vi "STED Control V18 DL.vi"() -> ()   [LabVIEW 2014]
uses:
  Controls/Button 2.ctl
  Type Defs/Image Acquisition Parameters.ctl
  Laser Controls.ctl
  Detectors.ctl
  Type Defs/P541.ctl
  Type Defs/M227.ctl
  Type Defs/P612.ctl
  Type Defs/M686.ctl
  Type Defs/P841.ctl
  Type Defs/ASI.ctl
  Type Defs/N664_V2.ctl
  Type Defs/STED Graph Controls.ctl
  Type Defs/Display Controls.ctl
  Type Defs/Z comp.ctl
  FPGA-7842R-Reference.ctl
  Manual Controls V2.ctl
  Scan Parameters.ctl
  <vilib>/Utility/miscctls.llb/LVPositionTypeDef.ctl
  Controls/StageStates.ctl
  DM_Dual_V2/Controls/Standard Action.ctl
  Focus Lock/Controls/Counter Action.ctl
  Focus Lock/Controls/Standard Action for Focus Lock.ctl
  <vilib>/Utility/miscctls.llb/LVRectTypeDef.ctl
  <vilib>/event_ctls.llb/lveventtype.ctl
  <vilib>/Utility/file.llb/Read From Spreadsheet File (DBL).vi
  <vilib>/FPGAPlugInAG/PCIe-7841R/niLvFpga_Open_PCIe-7841R.vi
  <vilib>/FPGAPlugInAG/PCIe-7841R/niLvFpga_Abort_PCIe-7841R.vi
  <vilib>/Utility/file.llb/Write To Spreadsheet File (DBL).vi
  <vilib>/rvi/interface/nirviOpenFPGA/nirviOpenFPGA.xnode
  FPGA Bitfiles/MainSTEDFPGAProj_FPGATarget_WaveformandLaser_sIm2Xng7ncM.lvbitx
  FPGA Target VIs/FPGA-7841R/Waveform and Laser Controls V7.vi
  <vilib>/rvi/interface/nirviMethod/nirviMethod.xnode
panel:
  in  "Wake Up FPGA":bool
  in  "z Comp.":T1
  out "Graph Ref Out":refnum<vi>[](array[refnum])
  out "Frame Counter":i32
  in  "Follow Cursor":bool
  in  "Laser Controls 2":T2={"Laser On Time (Ticks)"=16, "Laser Delay (Ticks)"=3}
  out "Channel 6":sgl[][](graph)
  out "Channel 5":sgl[][](graph)
  out "Channel 4":sgl[][](graph)
  out "Channel 3":sgl[][](graph)
  out "Channel 2":sgl[][](graph)
  out "Channel 1":sgl[][](graph)
  in  "Display Controls":T3
  in  "Graph Tools":T4={"Zoom Out"=FALSE, "Zoom In"=FALSE, "Reset Zoom"=FALSE, "Pan Tool"=FALSE, "Show Cursor"=FALSE, "Load File"=FALSE, "Fit Tool"=FALSE, "Smooth Tool"=FALSE, "Merge Tool"=FALSE, "Auto Scale"=FALSE, "Apply Color"=FALSE, "Color Map"=enum."Fire"}
  in  "Shutters":T5
  in  "Upper Objective Z - N664":T6={"Up N664"=FALSE, "Down N664"=FALSE, "Step Size (um)"=0.001, "Position (mm)"=0.0, "Home"=FALSE, "Save"=FALSE} {"Step Size (um)" min=0.001}
  in  "Cavity Translation Z - ASI":T7={"Up ASI"=FALSE, "Down ASI"=FALSE, "Step Size (um)"=0.001, "Z (um)"=0.001, "F (um)"=0.001, "Velocity"=0.001} caption="ASI" {"Velocity" min=0.001; "F (um)" min=0.001; "Z (um)" min=-1500.0 max=1500.0; "Step Size (um)" min=0.001}
  in  "Phase Comp Mirror - P841":T8={"Position (µm)"=0.0, "Step Size (µm)"=0.05, "Up P841"=FALSE, "Down P841"=FALSE}
  in  "Sample Stage XY - M686":T9={"Home Button"=FALSE, "Left Button"=FALSE, "Down Button"=FALSE, "Right Button"=FALSE, "Up Button"=FALSE, "X"=0.0, "Y"=0.0, "Step Size (um)"=1.0} {"Y" format="%#_8g"; "X" format="%#_8g"}
  in  "Bottom Objective XY - P612":T10
  in  "Abort AllStage":bool
  in  "Stages":T11={"M227"=TRUE, "N664"=TRUE, "P612"=TRUE, "M686"=TRUE, "P841"=TRUE, "ASI"=FALSE}
  in  "Sample Z Coarse - M227":T12
  in  "Tab Control":T13(tab)
  in  "SLM":T14
  in  "DM":T14
  in  "Timing":T14
  in  "Focus Lock":T14
  in  "Sequence":T14
  in  "Stage Monitor":T14
  in  "Camera":T14
  in  "Sequence Cluster":T15
  in  "Sample Z - P541":T16={"Step Up"=FALSE, "Step Down"=FALSE, "Z Position"=0.0, "Step Size (um)"=1.0, "Home"=FALSE, "Save"=FALSE}
  in  "Detectors":T17={"PMT"=TRUE, "Far Red (685/40 nm)"=FALSE, "Orange (624/40 nm)"=FALSE, "Green (525/50 nm)"=FALSE, "Sum All"=FALSE}
  in  "Laser Controls":T18 {"STED Power (V)" scale=0.0..10.0}
  in  "Save File Path":path=path "C:/isoSTED_Data/Temp/Test_0000.dbl"
  in  "Capture":bool
  in  "Image Acquisition Parameters":T19={"Scan Type"=enum."Beam Scanning", "Scan Mode"=enum."XY", "Fast Axis Frequency (Hz)"=15780.0, "Image Format"=256, "Line Accumulations"=100, "Frames Per Capture"=1, "Frames Accumulations"=1, "Image Dimension (um)"=[15.0, 15.0], "Number of Z Steps"=1, "Z Steps Size (um)"=1.0, "Pixel Size (nm)"=[58.59375, 58.59375], "Customized Image Format"=[]} {"Z Steps Size (um)" min=0.0; "Number of Z Steps" min=1; "Frames Accumulations" min=1; "Frames Per Capture" min=1; "Line Accumulations" min=1; "Image Format" items=["64 x 64"=64, "128 x 128"=128, "256 x 256"=256, "512 x 512"=512, "1024 x 1024"=1024, "2048 x 2048"=2048, "Customized..."=0]}
  in  "Live":T14
  in  "Exit":bool
  # "Piston"
  # "Defocus"
  # "Spherical"
  # "Frame Mode"
  # "Line Mode"
  # "Length"
  # "Height"
  # "XY"
  # "Z"
  # "Length"
  # "Height"
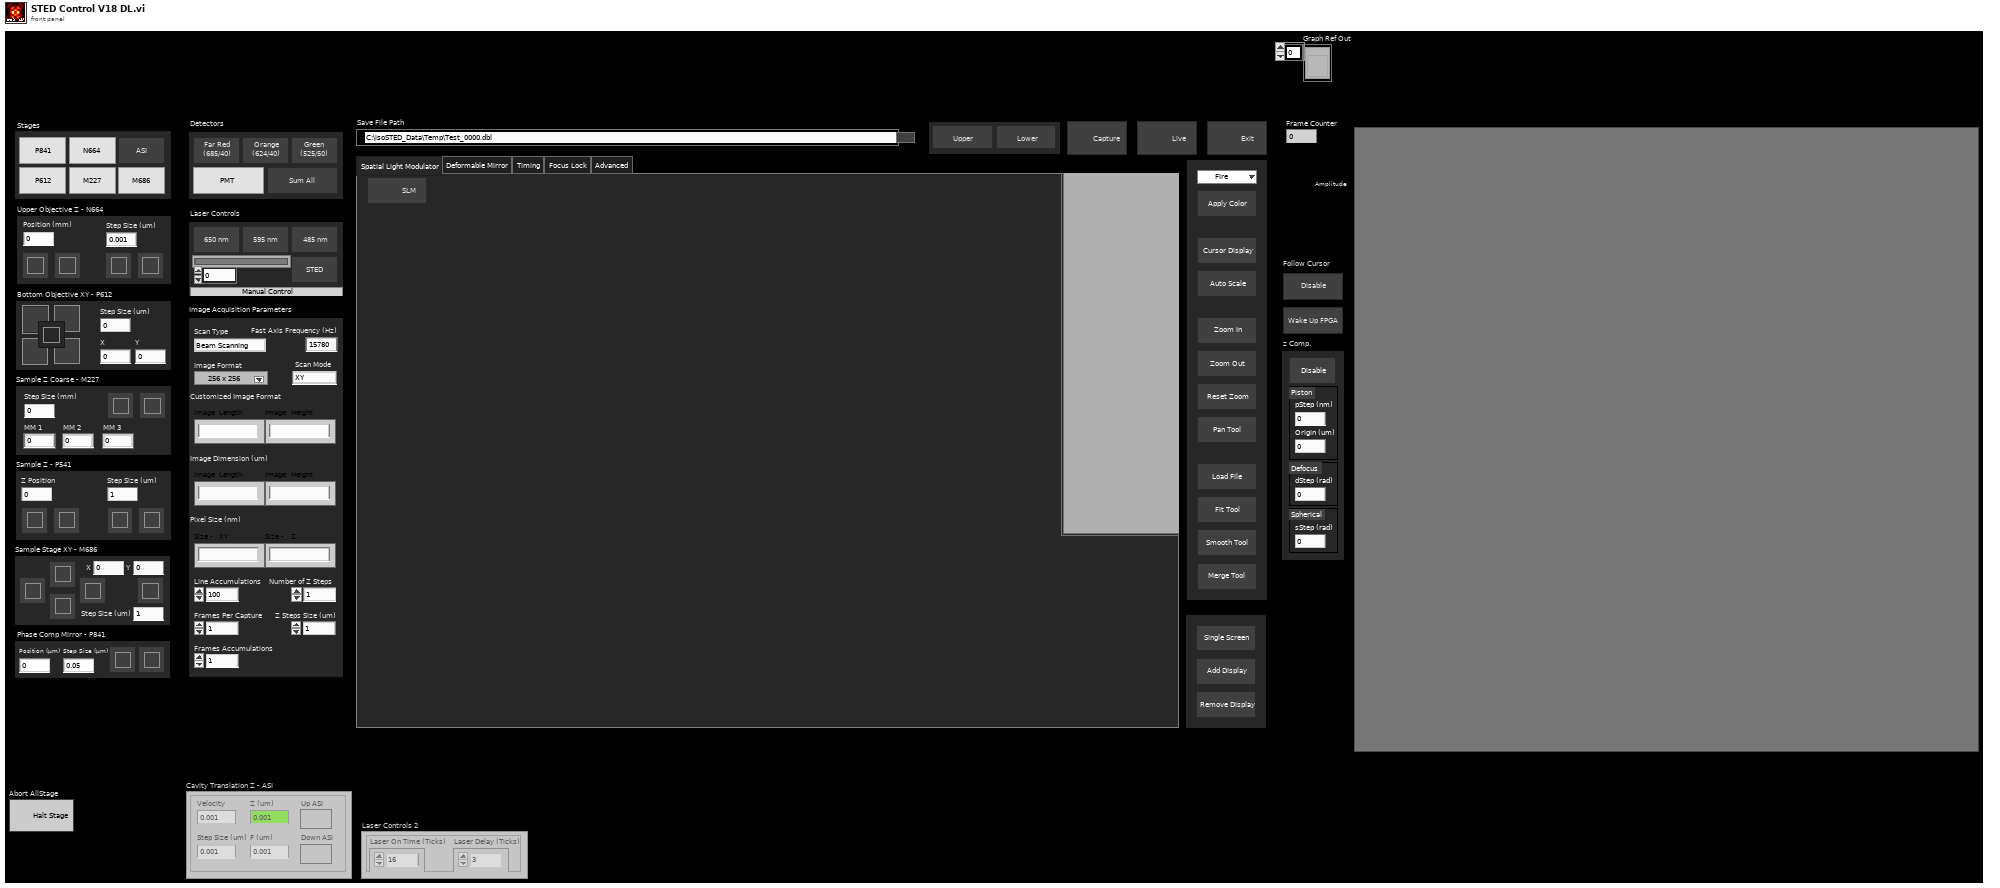
[diagram p1: front panel]
types:
  T1 = typedef "Z comp.ctl" = cluster{"Enable":bool, "pStep (nm)":dbl, "Origin (um)":dbl, "dStep (rad)":dbl, "sStep (rad)":dbl}
  T2 = cluster{"Laser On Time (Ticks)":i8, "Laser Delay (Ticks)":i8}
  T3 = typedef "Display Controls.ctl" = cluster{"Remove Display":bool, "Add Display":bool, "Single Screen":bool}
  T4 = typedef "STED Graph Controls.ctl" = cluster{"Zoom Out":bool, "Zoom In":bool, "Reset Zoom":bool, "Pan Tool":bool, "Show Cursor":bool, "Load File":bool, "Fit Tool":bool, "Smooth Tool":bool, "Merge Tool":bool, "Auto Scale":bool, "Apply Color":bool, "Color Map":enum16{"System", "Fire", "Gray", "Red", "Green", "Blue", "Cyan", "Magenta", "Yellow", "Red-White", "Green-White", "Blue-White", "Glow"}}
  T5 = cluster{"Upper Shutter":bool, "Lower Shutter":bool}
  T6 = typedef "N664_V2.ctl" = cluster{"Up N664":bool, "Down N664":bool, "Step Size (um)":dbl, "Position (mm)":dbl, "Home":bool, "Save":bool}
  T7 = typedef "ASI.ctl" = cluster{"Up ASI":bool, "Down ASI":bool, "Step Size (um)":dbl, "Z (um)":dbl, "F (um)":dbl, "Velocity":dbl}
  T8 = typedef "P841.ctl" = cluster{"Position (µm)":dbl, "Step Size (µm)":dbl, "Up P841":bool, "Down P841":bool}
  T9 = typedef "M686.ctl" = cluster{"Home Button":bool, "Left Button":bool, "Down Button":bool, "Right Button":bool, "Up Button":bool, "X":dbl, "Y":dbl, "Step Size (um)":dbl}
  T10 = typedef "P612.ctl" = cluster{"Home Button":bool, "Up Button":bool, "Left Button":bool, "Down Button":bool, "Right Button":bool, "Step Size (um)":dbl, "X":dbl, "Y":dbl}
  T11 = cluster{"M227":bool, "N664":bool, "P612":bool, "M686":bool, "P841":bool, "ASI":bool}
  T12 = typedef "M227.ctl" = cluster{"Up M227":bool, "Down M227":bool, "Step Size (mm)":dbl, "MM 1":dbl, "MM 2":dbl, "MM 3":dbl}
  T13 = enum32{"Spatial Light Modulator", "Deformable Mirror", "Timing", "Focus Lock", "Advanced"}
  T14 = typedef "Button 2.ctl" = bool
  T15 = cluster{"Operation Option":enum32{"frameSeq", "lineSeq"}, "AddSeq":bool, "DeleteSeq":bool, "DeleteAllSeq":bool, "Sequence List":enum32{"Seq 1", "Seq 2", "Seq 3", "Seq 4"}}
  T16 = typedef "P541.ctl" = cluster{"Step Up":bool, "Step Down":bool, "Z Position":dbl, "Step Size (um)":dbl, "Home":bool, "Save":bool}
  T17 = typedef "Detectors.ctl" = cluster{"PMT":bool, "Far Red (685/40 nm)":bool, "Orange (624/40 nm)":bool, "Green (525/50 nm)":bool, "Sum All":bool}
  T18 = typedef "Laser Controls.ctl" = cluster{"STED Power (V)":dbl, "STED":bool, "650 nm":bool, "590 nm":bool, "485 nm":bool, "Manual Control":bool}
  T19 = typedef "Image Acquisition Parameters.ctl" = cluster{"Scan Type":enum16{"Sample Scanning", "Beam Scanning"}, "Scan Mode":enum16{"XY", "XZ", "YZ", "XYZ"}, "Fast Axis Frequency (Hz)":dbl, "Image Format":u16, "Line Accumulations":u16, "Frames Per Capture":u16, "Frames Accumulations":u16, "Image Dimension (um)":dbl[], "Number of Z Steps":u16, "Z Steps Size (um)":dbl, "Pixel Size (nm)":dbl[], "Customized Image Format":dbl[]}
  T20 = typedef "Scan Parameters.ctl" = cluster{"Fast_Ax_Amp_V":dbl, "Fast_Ax_Off_V":dbl, "Slow_Ax_Amp_V":dbl, "Slow_Ax_Off_V ":dbl, "Slow_Ax_Max_V_VperS":dbl, "Slow_Ax1_Del25ns":i32, "Slow_Ax2_Del25ns":i32, "Stage_X_Off_V":dbl, "Stage_Y_Off_V":dbl, "Stage_Z_Off_V":dbl, "Galvo1_Off_V":dbl, "Galvo2_Off_V":dbl, "Last_Scan_Mode":enum16{"XY", "XZ", "YZ", "XYZ"}, "Current_Scan_Mode":enum16{"XY", "XZ", "YZ", "XYZ"}, "Fly_Back_Lines":u16, "Linear_Ramp_End":u32, "Z_Step_I16":i16, "Z_Start_I16":i16, "Laser_States _U32":u32, "590_Voltage_I16":i16, "775_AOM_Volt_I16":i16, "Blanking OFF":bool, "Unused_Axis_I16":i16}
  T21 = typedef "Manual Controls V2.ctl" = cluster{"Galvo 1 Position (I16)":i16, "Galvo 2 Position (I16)":i16, "X Axis Voltage (I16)":i16, "Y Axis Voltage (I16)":i16, "Z Axis Voltage (I16)":i16, "Res Mirror Amp (I16)":i16, "Res Mirror Mute":bool, "Upper Shutter":bool, "Lower Shutter":bool}
  T22 = typedef "FPGA-7842R-Reference.ctl" = enum16{"Stage Control", "Laser Control", "Unused Axis I16", "Exit", "Set Res Mirror", "Set Galvo", "Current Frame for Capture", "Default", "Close FPGA", "Stop Waveforms", "Start Waveforms", "Shutter Control", "Initialize"}
  T23 = typedef "Counter Action.ctl" = enum16{"Zero", "Plus One", "Read"}
  T24 = typedef "StageStates.ctl" = enum16{"POSITION", "MVR", "MOVE", "HALT", "ONTARGET", "ERROR", "EXIT", "HOME", "ZEROPOS", "NANOPOS", "QUIT", "ANALOG"}
  T25 = enum8{"Enabled", "Disabled", "Disabled and Grayed Out"}
  T26 = typedef "Standard Action.ctl" = enum16{"Read", "Write"}
  T27 = typedef "Standard Action for Focus Lock.ctl" = enum16{"Read", "Write"}
  T28 = typedef "LVRectTypeDef.ctl" = cluster{"Left":i16, "Top":i16, "Right":i16, "Bottom":i16}
  T29 = enum32{"Invalid", "Standard", "Closed", "Hidden", "Minimized", "Maximized"}
  T30 = typedef "lveventtype.ctl" = enum32{"Null", "Timeout", "Annotation Menu Selection", "Annotation Menu Selection?", "App Instance Close", "App Instance Close?", "Autoscale Range Change", "Bookmark Info Change", "Cell Edit", "Cell Edit?", "Cursor Grab", "Cursor Grab?", "Cursor Menu Selection", "Cursor Menu Selection?", "Cursor Move", "Cursor Release", "Data Change", "Direction Change", "Display State Change", "Drag Ended", "Drag Enter", "Drag Leave", "Drag Over", "Drag Source Update", "Drag Starting", "Drag Starting?", "Drop", "Exec State Change", "Key Down", "Key Down?", "Key Repeat", "Key Repeat?", "Key Up", "Listbox Double Click", "Menu Activation?", "Menu Selection (App)", "Menu Selection? (App)", "Menu Selection (User)", "Mouse Down", "Mouse Down?", "Mouse Enter", "Mouse Leave", "Mouse Move", "Mouse Up", "Mouse Wheel", "NI Security User Change (App)", "Pane Size", "Panel Close", "Panel Close?", "Panel Resize", "Plot Attribute Change", "Scale Range Change", "Shortcut Menu Activation?", "Shortcut Menu Selection (App)", "Shortcut Menu Selection? (App)", "Shortcut Menu Selection (User)", "Tree Double Click", "Tree Drag", "Tree Drag?", "Tree Drop", "Tree Drop?", "Tree Item Close", "Tree Item Close?", "Tree Item Open", "Tree Item Open?", "User Event", "Value Change"}
  T31 = typedef "LVPositionTypeDef.ctl" = cluster{"Left":i32, "Top":i32}
  T32 = cluster{"Upper Shutter":bool, "Upper Shutter":bool}
  T33 = cluster{bool, bool, dbl, "Numeric":dbl, "Numeric":dbl, "Numeric":dbl}
  T34 = cluster{"Down_N664":bool, "Down_N664":bool, "Step Size (um)":dbl, "Numeric":dbl, bool, bool}
  T35 = cluster{bool, bool, bool, bool, bool, dbl, "Numeric":dbl, "Numeric":dbl}
  T36 = cluster{bool, bool, bool, bool, bool, "Numeric":dbl, "Numeric":dbl, dbl}
  T37 = cluster{"Enable":bool, "pStep (nm)":bool, "Origin (um)":bool, "dStep (rad)":bool, "sStep (rad)":bool}
  T38 = typedef "MirrorModes_DUAL.ctl" = cluster{"Mode":string, "Amplitude":dbl}[][]
  T39 = cluster{"Detectors Parameters Out":T17, "Laser Parameters Out":T18, "Image Acquisition Parameters Out":T19}[]
  T40 = cluster{"Detectors Parameters Out":T17, "Laser Parameters Out":T18, "Image Acquisition Parameters Out":T19}
  T41 = cluster{"Scan Type":bool, "Scan Mode":bool, "Fast Axis Frequency (Hz)":bool, "Image Format":bool, "Line Accumulations":bool, "Frames Per Capture":bool, "Frames Accumulations":bool, "Image Dimension (um)":bool[], "Number of Z Steps":bool, "Z Steps Size (um)":bool, "Pixel Size (nm)":bool[], "Customized Image Format":bool[]}
  T42 = typedef "Focus Lock.ctl" = cluster{"EXIT":bool, "Lock Current":bool, "Manual":bool, "Drift":bool, "Move":bool, "Control Option":bool}
  T43 = typedef "LVAllMonitorsDisplayTypeDef.ctl" = cluster{"Bounds":cluster{"Left":i16, "Top":i16, "Right":i16, "Bottom":i16}, "Depth":i16}[]
  T44 = cluster{"Bounds":cluster{"Left":i16, "Top":i16, "Right":i16, "Bottom":i16}, "Depth":i16}
  T45 = enum16{"System", "Fire", "Gray", "Red", "Green", "Blue", "Cyan", "Magenta", "Yellow", "Red-White", "Green-White", "Blue-White", "Glow"}
  T46 = typedef "LVPointDoubleTypeDef.ctl" = cluster{"Cursor X":dbl, "Cursor Y":dbl}
  T47 = typedef "LVRangeTypeDef.ctl" = cluster{"Minimum":dbl, "Maximum":dbl, "Increment":dbl, "Minor Increment":dbl, "Start":dbl}
  T48 = cluster{"Operation Option":bool, "AddSeq":bool, "DeleteSeq":bool, "DeleteAllSeq":bool, "Sequence List":bool}
  T49 = typedef "IMAQ Image.ctl" = refnum<image>
  T50 = typedef "Waveform Data.ctl" = cluster{"Waveform Scan Parameters":cluster{"Scanning Mode":u8, "Fast Axis WF Length (Elements)":i32, "Fast Axis Sample Period (Ticks)":u32, "Slow Axis 1 WF Length (Elements)":i32, "Slow Axis 1 Sample Period (Ticks)":u32, "Slow Axis 1 Delay (25 ns) Steps":i32, "Slow Axis 2 WFLength (Elements)":i32, "Slow Axis 2 Sample Period (Ticks)":u32, "Slow Axis 2 Delay (25 ns) Steps":i32}, "Fast Axis Waveform":dbl[], "Slow Axis 1 Waveform":dbl[], "Slow Axis 2 Waveform":dbl[]}
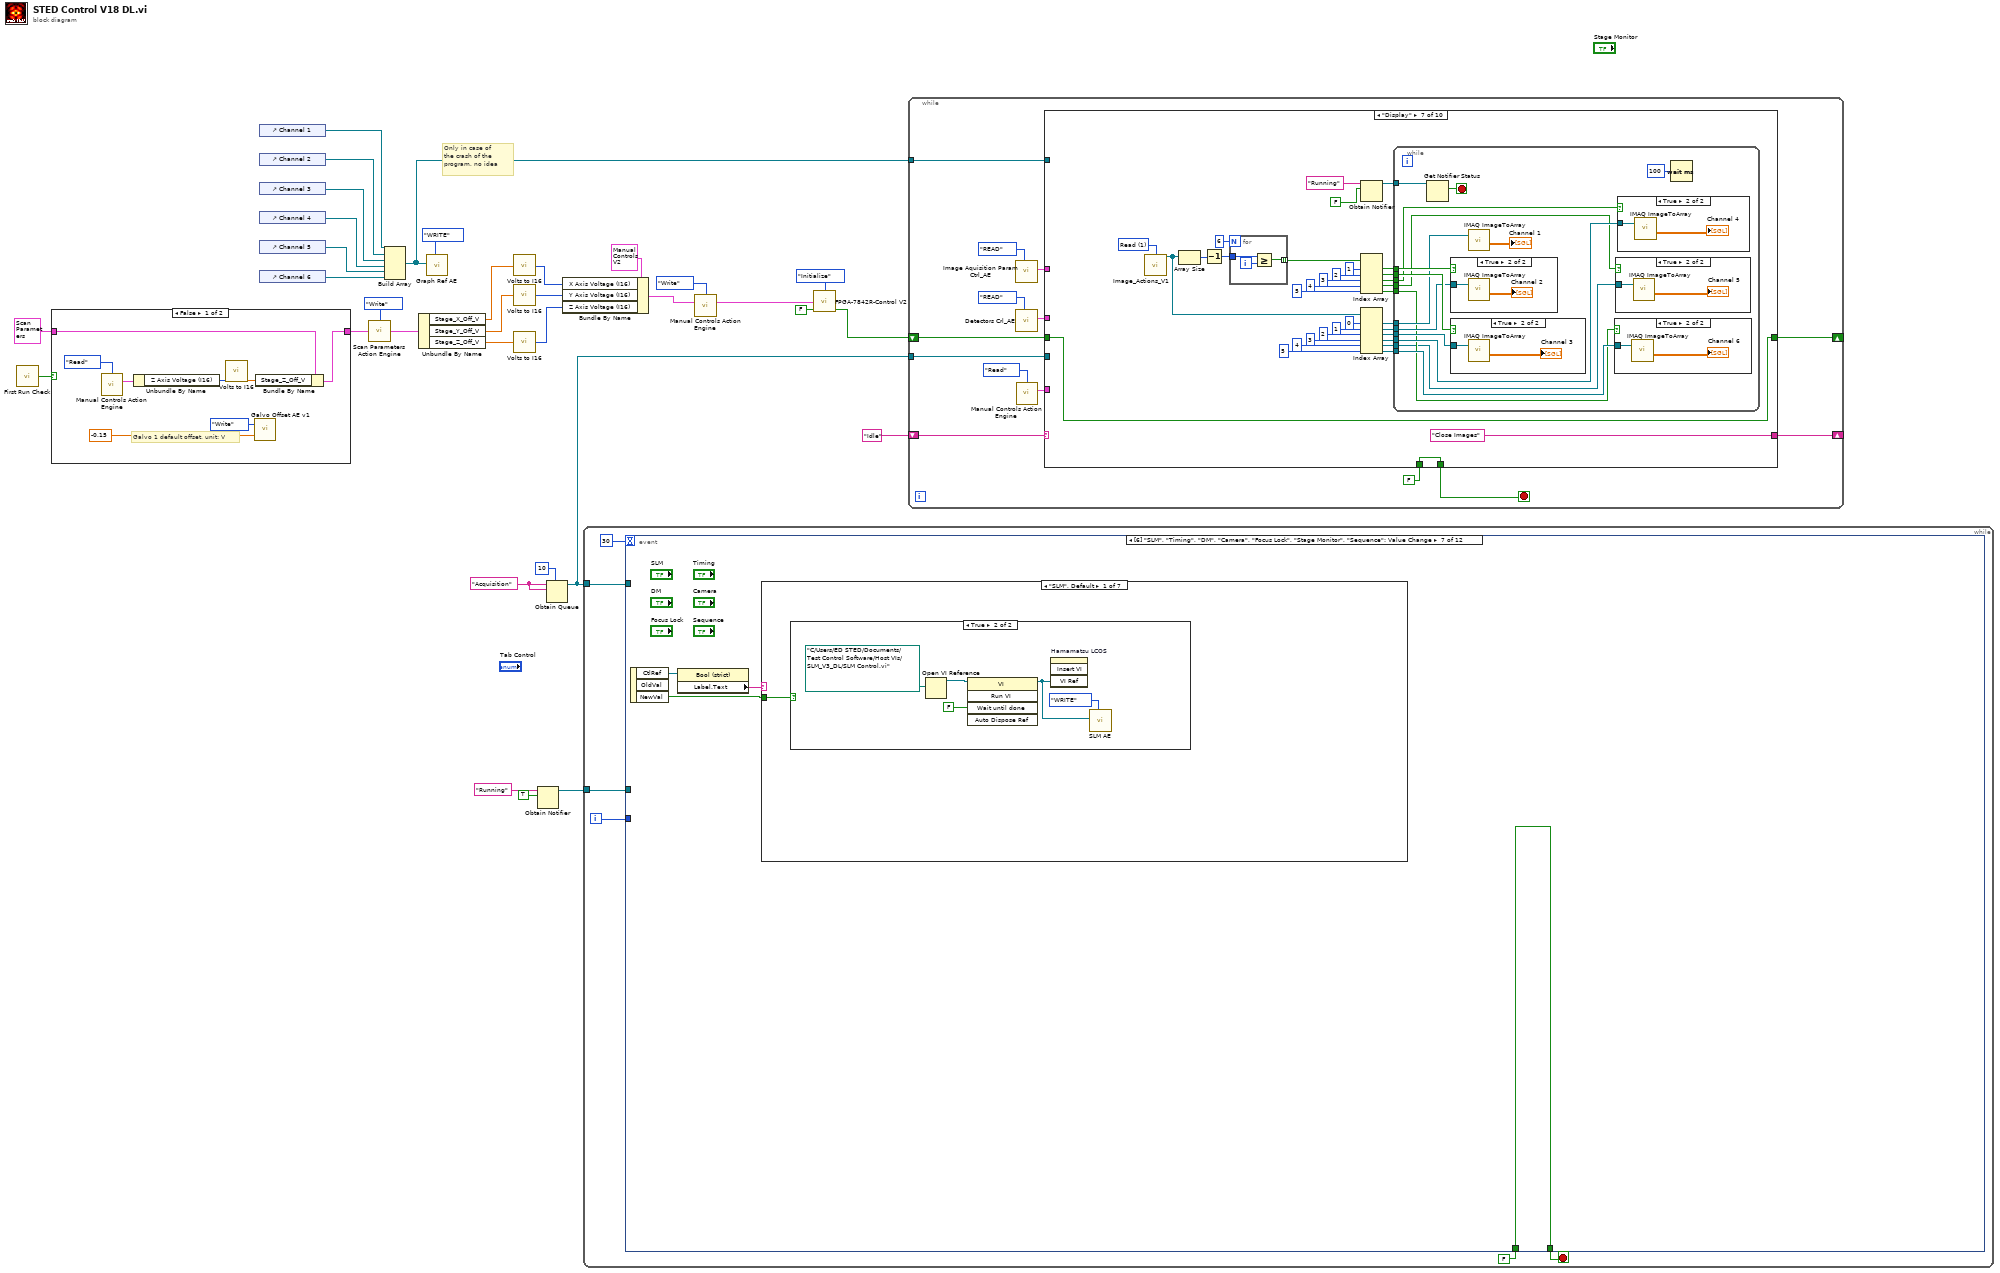
[diagram p0: block diagram]
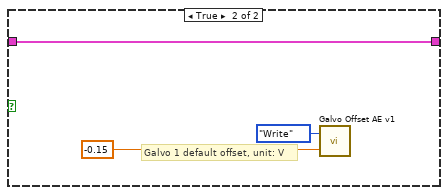
[diagram p2: hidden frame]
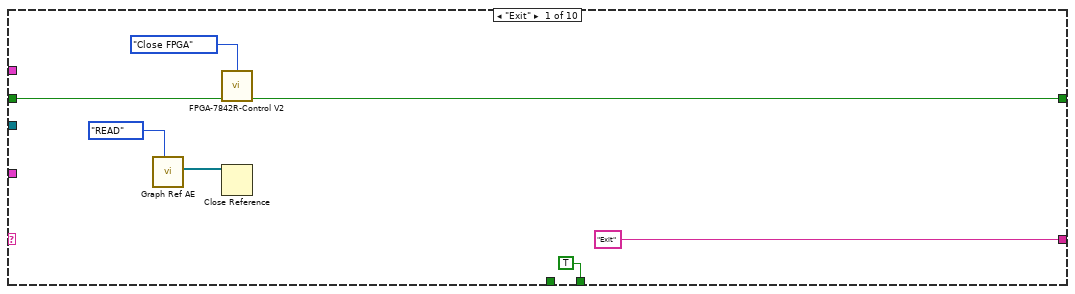
[diagram p3: hidden frame]
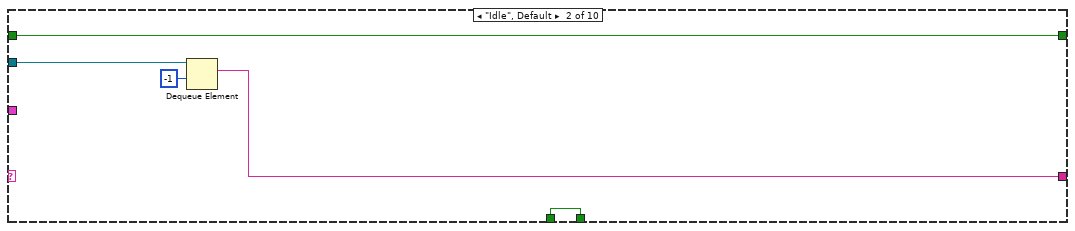
[diagram p4: hidden frame]
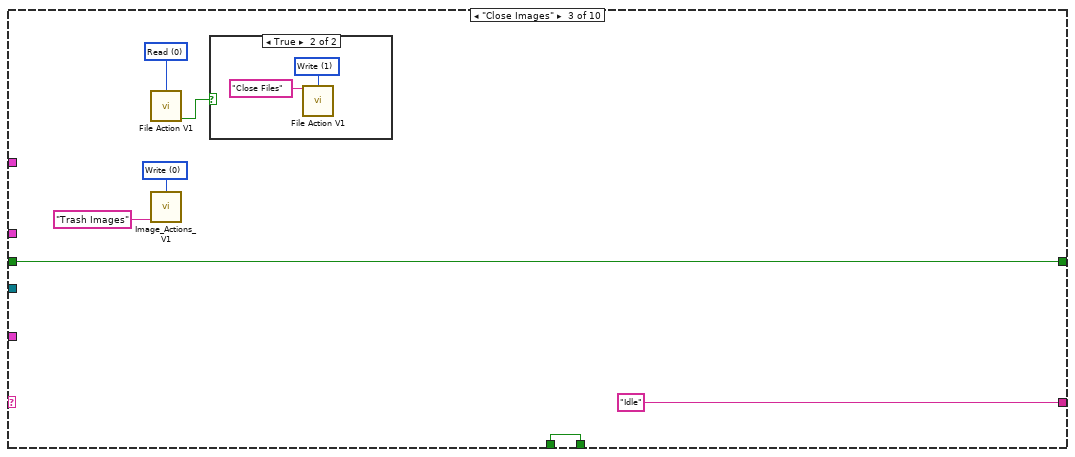
[diagram p5: hidden frame]
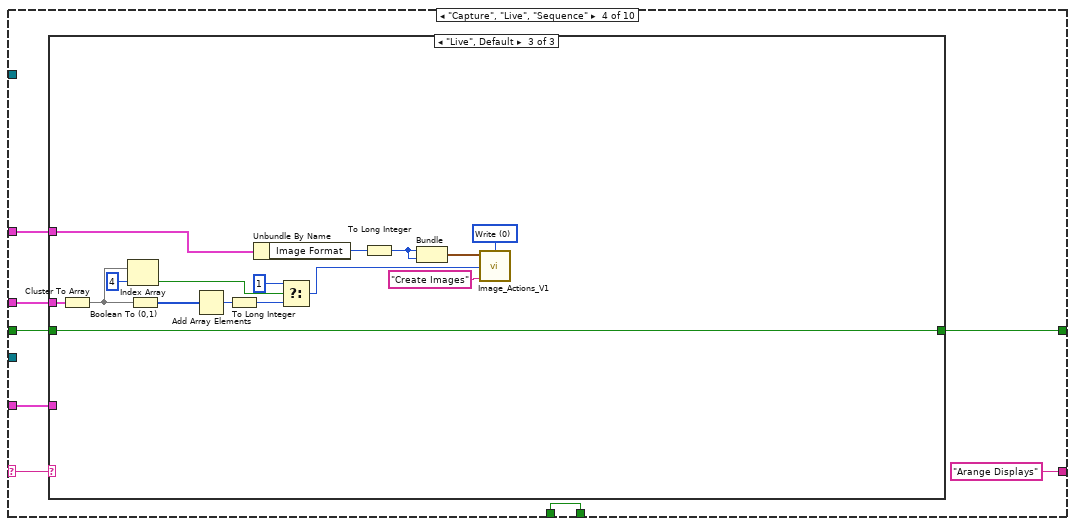
[diagram p7: hidden frame]
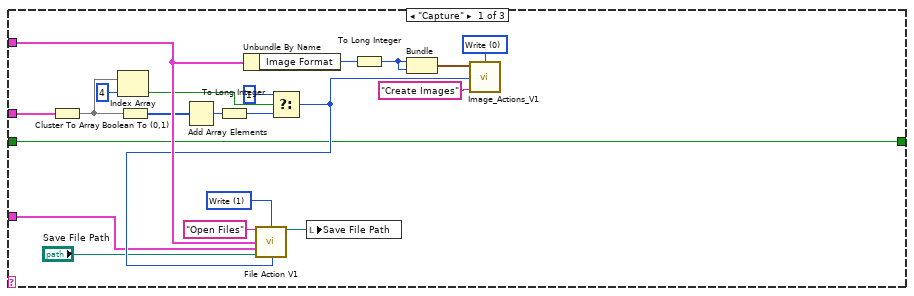
[diagram p8: hidden frame]
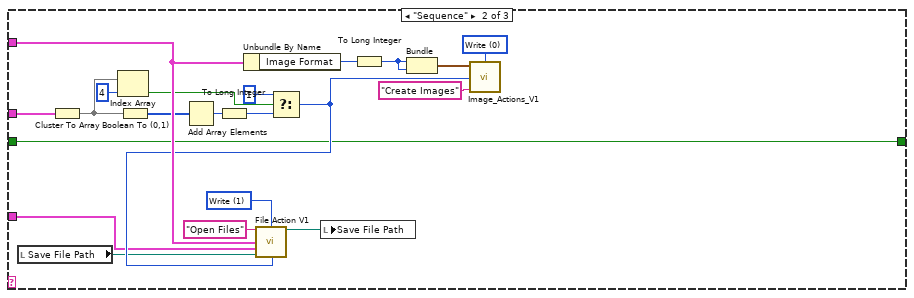
[diagram p9: hidden frame]
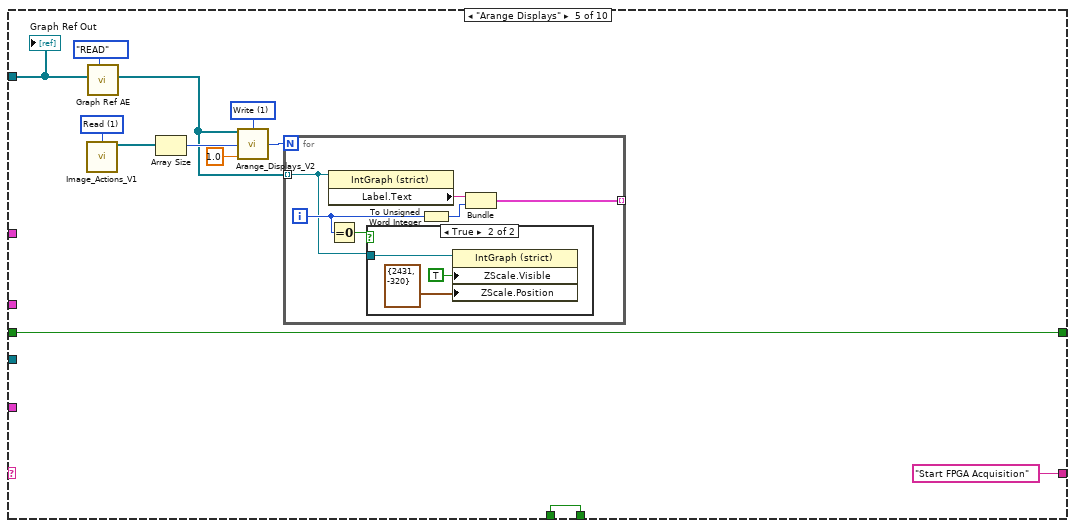
[diagram p10: hidden frame]
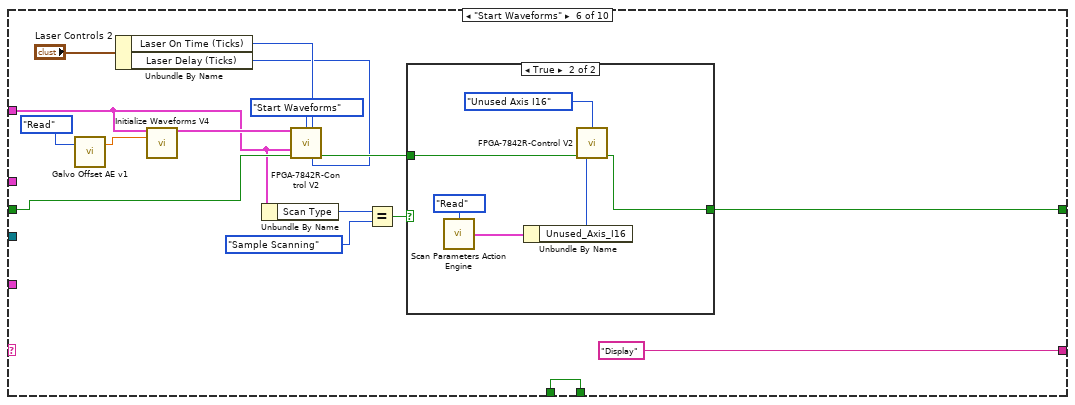
[diagram p12: hidden frame]
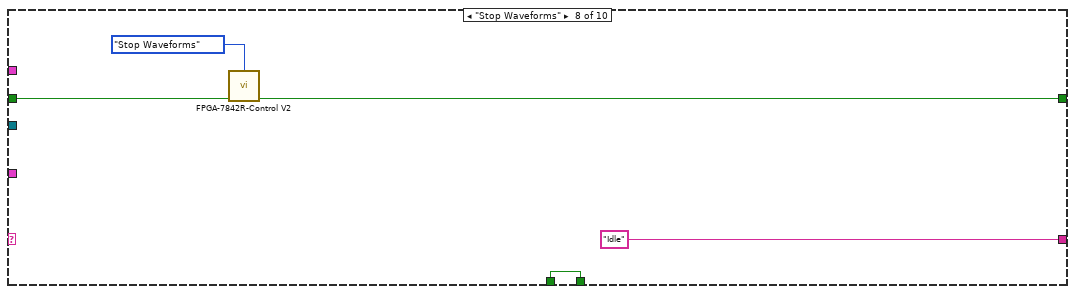
[diagram p19: hidden frame]
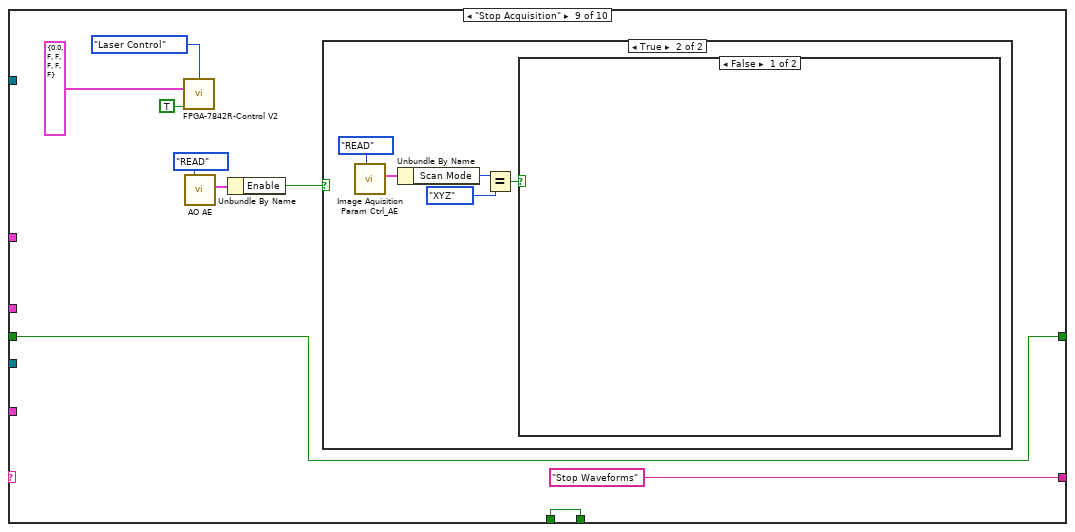
[diagram p20: hidden frame]
diagram:
  w16 = "Acquisition" ("name (unnamed)")
  # "Only in case of \nthe crash of the\nprogram, no idea"
  n1 = call "First Run Check.vi"() -> ("First Run?"=w10:bool)  [unwired: 15 in]
  n2 = case shown="False" w10 {
    tunnel: T20 {"Fast_Ax_Amp_V"=0.0, "Fast_Ax_Off_V"=0.0, "Slow_Ax_Amp_V"=0.0, "Slow_Ax_Off_V "=0.0, "Slow_Ax_Max_V_VperS"=0.0, "Slow_Ax1_Del25ns"=0, "Slow_Ax2_Del25ns"=0, "Stage_X_Off_V"=5.0, "Stage_Y_Off_V"=5.0, "Stage_Z_Off_V"=5.0, "Galvo1_Off_V"=0.0, "Galvo2_Off_V"=0.0, "Last_Scan_Mode"=enum."XY", "Current_Scan_Mode"=enum."XY", "Fly_Back_Lines"=0, "Linear_Ramp_End"=0, "Z_Step_I16"=0, "Z_Start_I16"=0, "Laser_States _U32"=0, "590_Voltage_I16"=0, "775_AOM_Volt_I16"=0, "Blanking OFF"=FALSE, "Unused_Axis_I16"=16384} ("Scan Parameters IN") -> [w41 w44]
    tunnel: [w36 w44] -> w8
    frame False {
      # "Galvo 1 default offset, unit: V"
      n3 = call "Manual Controls Action Engine.vi"("Action"=enum16{"Read", "Write"}."Read") -> ("Manual Controls Out"=w39:T21)  [unwired: 14 in]
      n4 = Unbundle By Name(w39) -> ("Z Axis Voltage (I16)"=w40:i16)
      n5 = call "Volts to I16.vi"("Volatge (I16)"=w40) -> ("Voltage (V)"=w37:dbl)  [unwired: 13 in, 1 out]
      n6 = call "Galvo Offset AE v1.vi"("Galvo 1 Offset In"=-0.15, "Action"=enum16{"Read", "Write"}."Write") -> ()  [unwired: 2 out]
      n7 = Bundle By Name(cluster=w41, "Stage_Z_Off_V"=w37) -> (w36:T20)
    }
    frame True {
      # "Galvo 1 default offset, unit: V"
      n8 = call "Galvo Offset AE v1.vi"("Galvo 1 Offset In"=-0.15, "Action"=enum16{"Read", "Write"}."Write") -> ()  [unwired: 2 out]
    }
  }
  n9 = control-ref of="Channel 1"() -> (w5:refnum<vi>)
  n10 = control-ref of="Channel 2"() -> (w6:refnum<vi>)
  n11 = control-ref of="Channel 3"() -> (w7:refnum<vi>)
  n12 = control-ref of="Channel 4"() -> (w2:refnum<vi>)
  n13 = control-ref of="Channel 5"() -> (w4:refnum<vi>)
  n14 = control-ref of="Channel 6"() -> (w3:refnum<vi>)
  n15 = call "Scan Parameters Action Engine.vi"("Action"=enum16{"Read", "Write"}."Write", "Scan Parameters IN"=w8) -> ("Scan Parameters OUT"=w26:T20)  [unwired: 13 in]
  n16 = Build Array(w5, w6, w7, w2, w4, w3) -> (w1:refnum<vi>[])
  n17 = Unbundle By Name(w26) -> ("Stage_X_Off_V"=w22:dbl, "Stage_Y_Off_V"=w21:dbl, "Stage_Z_Off_V"=w20:dbl)
  n18 = call "Graph Ref AE.vi"("Action"=enum16{"READ", "WRITE"}."WRITE", "Graph Ref In"=w1) -> ()  [unwired: 9 in, 1 out]
  n19 = call "Volts to I16.vi"("Voltage (V)"=w22) -> ("I16"=w23:i16)  [unwired: 13 in, 1 out]
  n20 = call "Volts to I16.vi"("Voltage (V)"=w21) -> ("I16"=w24:i16)  [unwired: 13 in, 1 out]
  n21 = call "Volts to I16.vi"("Voltage (V)"=w20) -> ("I16"=w25:i16)  [unwired: 13 in, 1 out]
  n22 = Obtain Notifier(name (unnamed)="Running", notification data type=TRUE) -> (notifier out=w12:refnum<notifier>)  [unwired: 2 in, 2 out]
  n23 = Obtain Queue(max queue size (-1, unlimited)=10, name (unnamed)=w16, element data type=w16) -> (queue out=w18:refnum<queue>)  [unwired: 2 in, 2 out]
  n24 = Bundle By Name(cluster=T21 {"Galvo 1 Position (I16)"=-280, "Galvo 2 Position (I16)"=0, "X Axis Voltage (I16)"=16384, "Y Axis Voltage (I16)"=16384, "Z Axis Voltage (I16)"=16384, "Res Mirror Amp (I16)"=0, "Res Mirror Mute"=FALSE, "Upper Shutter"=FALSE, "Lower Shutter"=FALSE} ("Manual Controls"), "X Axis Voltage (I16)"=w23, "Y Axis Voltage (I16)"=w24, "Z Axis Voltage (I16)"=w25) -> (w27:T21)
  n25 = while {
    tunnel: w18 -> [w48]
    tunnel: w12 -> [w45]
    i -> [w46]
    stop <- w50 stop-if-true
    n26 = event shown="[6] \"SLM\", \"Timing\", \"DM\", \"Camera\", \"Focus Lock\", \"Stage Monitor\", \"Sequence\": Value Change" {
      selector: _ -> [_ _ _ _ _ _ _ _ _ _ _ _]
      dyn-events: _ -> [_ _ _ _ _ _ _ _ _ _ _ _]
      timeout: 30 -> [_ _ _ _ _ _ _ _ _ _ _ _]
      tunnel: [w58 _ w265 w335 w469 _ w816 w915 w1133 w1160 _ w1289] -> w50
      tunnel: FALSE -> [w58 _ w265 w335 w469 _ w816 w915 w1133 w1160 _ _]
      tunnel: w48 -> [w55 _ w264 _ _ _ _ _ _ _ _ w1288]
      tunnel: w46 -> [w53 _ _ _ _ _ _ _ _ _ _ _]
      tunnel: w45 -> [w51 _ w262 _ _ _ _ _ _ _ _ w1282]
      event Timeout {
        n27 = event-data() -> ()  [unwired: 1 in, 3 out]
        n28 = Equal To 0?(x=w53) -> (x = 0?=w52:bool)
        n29 = Get Notifier Status(notifier=w51) -> (current notification=w57:bool)  [unwired: 1 in, 4 out]
        n30 = case shown="True" w52 {
          frame False {
            w68 = enum16{"WRITE", "READ", "HOME", "SAVE HOME"}."READ" ("Enum")
            n31 = call "AO AE.vi"("Action"=enum16{"READ", "WRITE"}."READ") -> ("Z Comp. Output"=w61:T1)  [unwired: 8 in, 2 out]
            n32 = Unbundle By Name(w61) -> ("Enable"=w66:bool, "Origin (um)"=w62:dbl, "pStep (nm)"=w63:dbl, "dStep (rad)"=w60:dbl, "sStep (rad)"=w59:dbl)
            n33 = call "Image Aquisition Param Ctrl_AE.vi"("Action"=enum16{"READ", "WRITE"}."READ") -> ("Image Acquisition Parameters Out"=w102:T19)  [unwired: 10 in]
            n34 = call "Detectors Crl_AE.vi"("Action"=enum16{"READ", "WRITE"}."READ") -> ("Detectors Parameters Out"=w103:T17)  [unwired: 10 in]
            n35 = call "LASERs_ Crl_AE.vi"("Action"=enum16{"READ", "WRITE"}."READ") -> ("Laser Parameters Out"=w104:T18)  [unwired: 10 in]
            n36 = local write "z Comp."(w61) -> ()
            n37 = local write "Image Acquisition Parameters"(w102) -> ()
            n38 = local write "Detectors"(w103) -> ()
            n39 = local write "Laser Controls"(w104) -> ()
            n40 = call "Frame Counter.vi"("Action"=Counter_Action."Read") -> ("Num"=w67:i32)
            "Frame Counter" <- w67
            n41 = case shown="False" w66 {
              tunnel: w67 -> [_ w108]
              tunnel: w63 -> [_ w109]
              tunnel: w62 -> [_ w107]
              tunnel: w61 -> [_ _]
              tunnel: w60 -> [_ w106]
              tunnel: w59 -> [_ w105]
              frame False {
              }
              frame True {
                n42 = local read "Capture"() -> (w116:bool)
                n43 = local read "Live"() -> (w117:T14)
                n44 = call "Image Aquisition Param Ctrl_AE.vi"("Action"=enum16{"READ", "WRITE"}."READ") -> ("Image Acquisition Parameters Out"=w118:T19)  [unwired: 10 in]
                n45 = Or(x=w116, y=w117) -> (x .or. y?=w113:T14)
                n46 = Unbundle By Name(w118) -> ("Scan Mode"=w115:enum16{"XY", "XZ", "YZ", "XYZ"}, "Number of Z Steps"=w110:u16)
                n47 = Equal?(x=enum16{"XY", "XZ", "YZ", "XYZ"}."XYZ", y=w115) -> (x = y?=w112:bool)
                n48 = And(x=w113, y=w112) -> (x .and. y?=w111:T14)
                n49 = case shown="True" w111 {
                  tunnel: w108 -> [_ w129]
                  tunnel: w110 -> [_ w128]
                  tunnel: w109 -> [_ w127]
                  tunnel: w107 -> [_ w126]
                  tunnel: w106 -> [_ w121]
                  tunnel: w105 -> [_ w120]
                  frame False {
                  }
                  frame True {
                    n50 = Quotient & Remainder(x=w129, y=w128) -> (x-y*floor(x/y)=w122:i32)  [unwired: 1 out]
                    n51 = control-ref of="Abort AllStage"() -> (w124:refnum<vi>)
                    n52 = call "Defocus and Spherical Comp V2.vi"("Spherical Step"=w120, "Defocus Step"=w121, "Step #"=w122) -> ()  [unwired: 1 in]
                    n53 = call "Piston Comp.vi"("Abort"=w124, "Step Size"=w127, "Step #"=w122, "Original Position"=w126, "Action"=enum16{"MOVE", "BACK TO ORIGINE"}."MOVE") -> ("position"=w123:dbl)  [unwired: 5 in]
                    n54 = property on="Position (µm)" class="DigNum (strict)"("Value"=w123) -> ()  [unwired: 2 in, 2 out]
                  }
                }
              }
            }
            n55 = call "Stage_position_ae.vi"("StageID"="M686", "Enum"=w68) -> ("Position Out"=w78:dbl[])  [unwired: 8 in, 1 out]
            n56 = call "Stage_position_ae.vi"("StageID"="M227", "Enum"=w68) -> ("Position Out"=w85:dbl[])  [unwired: 8 in, 1 out]
            n57 = call "Stage_position_ae.vi"("StageID"="N664", "Enum"=w68) -> ("Position Out"=w71:dbl[])  [unwired: 8 in, 1 out]
            n58 = call "Stage_position_ae.vi"("StageID"="P841", "Enum"=w68) -> ("Position Out"=w92:dbl[])  [unwired: 8 in, 1 out]
            n59 = call "Stage_position_ae.vi"("StageID"="P612", "Enum"=w68) -> ("Position Out"=w69:dbl[])  [unwired: 8 in, 1 out]
            n60 = Index Array(array=w71, index=0) -> (element=w88:dbl)
            n61 = Index Array(array=w92, index=0) -> (element=w65:dbl)
            n62 = Index Array(array=w69, index #1=0 ("index"), index #2=1 ("index"), index #3=2 ("index")) -> (element #1=w98:dbl, element #2=w95:dbl, element #3=w93:dbl)
            n63 = Index Array(array=w78, index #1=0 ("index"), index #2=1 ("index")) -> (element #1=w75:dbl, element #2=w74:dbl)
            n64 = Index Array(array=w85, index #1=0 ("index"), index #2=1 ("index"), index #3=2 ("index")) -> (element #1=w82:dbl, element #2=w81:dbl, element #3=w80:dbl)
            n65 = property on="Position (µm)" class="DigNum (strict)"("Value"=w65) -> ()  [unwired: 2 in, 2 out]
            n66 = property on="Position (mm)" class="DigNum (strict)"("Value"=w88) -> ()  [unwired: 2 in, 2 out]
            n67 = property on="X" class="DigNum (strict)"("Value"=w98) -> ()  [unwired: 2 in, 2 out]
            n68 = property on="Y" class="DigNum (strict)"("Value"=w95) -> ()  [unwired: 2 in, 2 out]
            n69 = property on="X" class="DigNum (strict)"("Value"=w75) -> ()  [unwired: 2 in, 2 out]
            n70 = property on="MM 1" class="DigNum (strict)"("Value"=w82) -> ()  [unwired: 2 in, 2 out]
            n71 = property on="MM 2" class="DigNum (strict)"("Value"=w81) -> ()  [unwired: 2 in, 2 out]
            n72 = property on="Z Position" class="DigNum (strict)"("Value"=w93) -> ()  [unwired: 2 in, 2 out]
            n73 = property on="Y" class="DigNum (strict)"("Value"=w74) -> ()  [unwired: 2 in, 2 out]
            n74 = property on="MM 3" class="DigNum (strict)"("Value"=w80) -> ()  [unwired: 2 in, 2 out]
          }
          frame True {
            w130 = T25."Disabled and Grayed Out" ("Disabled")
            w131 = FALSE ("SLM")
            w134 = enum16{"WRITE", "READ", "HOME", "SAVE HOME"}."SAVE HOME" ("Enum")
            w146 = FALSE ("Upper Shutter")
            n75 = local read "Image Acquisition Parameters"() -> (w153:T19)
            n76 = local read "Laser Controls"() -> (w151:T18)
            n77 = local read "Detectors"() -> (w150:T17)
            n78 = Bundle("Upper Shutter"=w146, "Upper Shutter"=w146) -> (w147:T32)  [unwired: 1 in]
            n79 = property on="Shutters" class="Clust (strict)"("Value"=w147) -> ()  [unwired: 2 in, 2 out]
            n80 = call "Image Aquisition Param Ctrl_AE.vi"("Action"=enum16{"READ", "WRITE"}."WRITE", "Image Acquisition Parameters In"=w153) -> ()  [unwired: 9 in, 1 out]
            n81 = call "Detectors Crl_AE.vi"("Action"=enum16{"READ", "WRITE"}."WRITE", "Detectors Parameters In"=w150) -> ()  [unwired: 9 in, 1 out]
            n82 = call "LASERs_ Crl_AE.vi"("Action"=enum16{"READ", "WRITE"}."WRITE", "Laser Parameters In"=w151) -> ()  [unwired: 9 in, 1 out]
            n83 = property on="Stages" class="Clust (strict)"() -> ("Controls[]"=w148:refnum<vi>[])  [unwired: 2 in, 2 out]
            n84 = for {
              tunnel: w148 -> [w158] mode=indexing
              n85 = property class="Ctl"(reference=w158) -> ("Label.Text"=w156:string, "Value"=w160:variant)  [unwired: 1 in, 2 out]
              n86 = Variant To Data(type=TRUE, Variant=w160) -> (data=w157:bool)  [unwired: 1 in, 1 out]
              n87 = call "All_Stages_Aloha.vi"("Aloha"=w157, "Stage ID"=w156) -> ("Position Out"=w155:dbl[])  [unwired: 9 in]
              n88 = case shown="\"M686\"" w156 {
                tunnel: w155 -> [_ w167 w175 w182 w191 w202 w212]
                frame "0", Default {
                }
                frame "M227" {
                  w171 = FALSE
                  n89 = Index Array(array=w167, index #1=0 ("index"), index #2=1 ("index"), index #3=2 ("index")) -> (element #1=w163:dbl, element #2=w162:dbl, element #3=w161:dbl)
                  n90 = Bundle(w171, w171, 0.0, "Numeric"=w163, "Numeric"=w162, "Numeric"=w161) -> (w169:T33)  [unwired: 1 in]
                  n91 = To Variant(anything=w169) -> (Variant=w168:variant)
                  n92 = property on="Sample Z Coarse - M227" class="Clust"("Value"=w168) -> ()  [unwired: 2 in, 2 out]
                }
                frame "N664" {
                  w172 = FALSE
                  w178 = FALSE ("Down_N664")
                  n93 = Index Array(array=w175, index=0) -> (element=w176:dbl)
                  n94 = Bundle("Down_N664"=w178, "Down_N664"=w178, "Step Size (um)"=1.0, "Numeric"=w176, w172, w172) -> (w174:T34)  [unwired: 1 in]
                  n95 = To Variant(anything=w174) -> (Variant=w173:variant)
                  n96 = property on="Upper Objective Z - N664" class="Clust"("Value"=w173) -> ()  [unwired: 2 in, 2 out]
                }
                frame "P612" {
                  w190 = FALSE
                  n97 = Index Array(array=w182, index #1=0, index #2=1, index #3=2 ("index")) -> (element #1=w187:dbl, element #2=w185:dbl, element #3=w180:dbl)
                  n98 = Bundle(w190, w190, w190, w190, w190, 1.0, "Numeric"=w187, "Numeric"=w185) -> (w186:T35)  [unwired: 1 in]
                  n99 = To Variant(anything=w186) -> (Variant=w181:variant)
                  n100 = property on="Bottom Objective XY - P612" class="Clust"("Value"=w181) -> ()  [unwired: 2 in, 2 out]
                  n101 = property on="Z Position" class="DigNum (strict)"("Value"=w180) -> ()  [unwired: 2 in, 2 out]
                }
                frame "M686" {
                  w200 = FALSE
                  n102 = Index Array(array=w191, index #1=0, index #2=1) -> (element #1=w195:dbl, element #2=w194:dbl)
                  n103 = Bundle(w200, w200, w200, w200, w200, "Numeric"=w195, "Numeric"=w194, 1.0) -> (w198:T36)  [unwired: 1 in]
                  n104 = To Variant(anything=w198) -> (Variant=w196:variant)
                  n105 = property on="Sample Stage XY - M686" class="Clust"("Value"=w196) -> ()  [unwired: 2 in, 2 out]
                  n106 = call "M686_timer.vi"("Reset"=TRUE) -> ()  [unwired: 1 out]
                }
                frame "P841" {
                  n107 = Index Array(array=w202, index=0) -> (element=w201:dbl)
                  n108 = property on="Position (µm)" class="DigNum (strict)"("Value"=w201) -> ()  [unwired: 2 in, 2 out]
                }
                frame "ASI" {
                  w208 = FALSE
                  n109 = Add Array Elements(numeric array=w212) -> (sum=w214:dbl)
                  n110 = Index Array(array=w212, index #1=0 ("index"), index #2=1 ("index")) -> (element #1=w207:dbl, element #2=w206:dbl)
                  n111 = Divide(x=w214, y=2000.0) -> ()  [unwired: 1 out]
                  n112 = Bundle By Name(cluster=T7 {"Up ASI"=FALSE, "Down ASI"=FALSE, "Step Size (um)"=0.001, "Z (um)"=0.001, "F (um)"=0.001, "Velocity"=0.001} ("Cavity Translation Z - ASI"), "Up ASI"=w208, "Down ASI"=w208, "Step Size (um)"=1.0, "Z (um)"=w207, "F (um)"=w206, "Velocity"=0.1) -> (w204:T7)
                  n113 = To Variant(anything=w204) -> (Variant=w205:variant)
                  n114 = property on="Cavity Translation Z - ASI" class="Clust"("Value"=w205) -> ()  [unwired: 2 in, 2 out]
                }
              }
            }
            n115 = call-poly <vilib>:"Read From Spreadsheet File.vi"("format (%.3f)"="%.4f", "number of rows (all:-1)"=1, "file path (dialog if empty)"=path "C:/Users/ED STED/Documents/Test Control Software/Host VIs/Stages/Stage Positions/home position.csv") -> ("first row"=w143:dbl[])  [unwired: 4 in, 4 out]
            n116 = Index Array(array=w143, index #1=0 ("index"), index #2=1 ("index")) -> (element #1=w139:dbl, element #2=w140:dbl)
            n117 = Build Array(w139) -> (w138:dbl[])
            n118 = Build Array(w140) -> (w136:dbl[])
            n119 = call "Stage_position_ae.vi"("Position In"=w138, "StageID"="P541", "Enum"=w134) -> ()  [unwired: 7 in, 2 out]
            n120 = call "Stage_position_ae.vi"("Position In"=w136, "StageID"="N664", "Enum"=w134) -> ()  [unwired: 7 in, 2 out]
            n121 = local write "Sequence"(w131) -> ()
            n122 = local write "Focus Lock"(w131) -> ()
            n123 = local write "SLM"(w131) -> ()
            n124 = local write "Timing"(w131) -> ()
            n125 = local write "DM"(w131) -> ()
            n126 = local write "Camera"(w131) -> ()
            n127 = property on="Sequence Cluster" class="Clust"("DisabledEnum"=w130) -> ()  [unwired: 2 in, 2 out]
            n128 = property on="Sequence List" class="RadioBtnsControl (strict)"("DisabledEnum"=w130) -> ()  [unwired: 2 in, 2 out]
            n129 = property on="Seq 3" class="Bool (strict)"("DisabledEnum"=w130) -> ()  [unwired: 2 in, 2 out]
            n130 = property on="Seq 1" class="Bool (strict)"("DisabledEnum"=w130) -> ()  [unwired: 2 in, 2 out]
            n131 = property on="Seq 2" class="Bool (strict)"("DisabledEnum"=w130) -> ()  [unwired: 2 in, 2 out]
            n132 = property on="Seq 4" class="Bool (strict)"("DisabledEnum"=w130) -> ()  [unwired: 2 in, 2 out]
            n133 = call "Frame Counter.vi"("Action"=Counter_Action."Zero") -> ()  [unwired: 1 out]
          }
        }
        n134 = local read "Capture"() -> (w56:bool)
        n135 = And(x=w57, y=w56) -> (x .and. y?=w54:bool)
        n136 = case shown="True" w54 {
          tunnel: w55 -> [_ w220]
          frame False {
          }
          frame True {
            w218 = T25."Enabled" ("Disabled")
            n137 = local write "Capture"(FALSE ("Capture")) -> ()
            n138 = call "Frame Counter.vi"("Action"=Counter_Action."Zero") -> ()  [unwired: 1 out]
            n139 = Enqueue Element(queue=w220, element="Stop Acquisition" ("f")) -> ()  [unwired: 2 in, 3 out]
            n140 = property on="Live" class="Bool (strict)"("DisabledEnum"=w218) -> ()  [unwired: 2 in, 2 out]
            n141 = property on="Exit" class="Bool"("DisabledEnum"=w218) -> ()  [unwired: 2 in, 2 out]
          }
        }
      }
      event Value Change {
        w229 = Standard_Action."Read" ("Action")
        n142 = event-data() -> ("NewVal"=w230:T1, "OldVal"=w235:T1)  [unwired: 1 in]
        n143 = Not Equal?(x=w230, y=w235) -> (x != y?=w234:T37)
        n144 = Unbundle By Name(w230) -> ("Enable"=w233:bool)
        n145 = Unbundle By Name(w234) -> ("Enable"=w232:bool)
        n146 = call "Pixel Value (-1 to 1) DUAL AE.vi"("Action"=w229) -> ("Pixel Value (-1 to 1) Out"=w222:dbl[][])  [unwired: 14 in]
        n147 = call "Mirror_Mode_DUAL_AE.vi"("Action"=w229) -> ("Mirror Modes Out"=w228:T38)  [unwired: 14 in]
        n148 = And(x=w233, y=w232) -> (x .and. y?=w231:bool)
        n149 = case shown="False" w231 {
          tunnel: w230 -> [w239 w248]
          tunnel: w222 -> [w236 w241]
          tunnel: w228 -> [w240 w242]
          tunnel: [w237 w243] -> w227
          tunnel: [w239 w243] -> w225
          tunnel: [w236 w241] -> w224
          tunnel: [w240 w242] -> w223
          frame False {
            n150 = Bundle By Name(cluster=w239, "Origin (um)"=0.0) -> (w237:T1)
          }
          frame True {
            n151 = call "AE_AllStages_Action V2.vi"("Stage ID"="P841" ("StageID"), "Action"=StageStates."MVR") -> ("Position Out"=w244:dbl[])  [unwired: 7 in, 2 out]
            n152 = Index Array(array=w244, index=0) -> (element=w247:dbl)
            n153 = Bundle By Name(cluster=w248, "Origin (um)"=w247) -> (w243:T1)
          }
        }
        n154 = local write "z Comp."(w227) -> ()
        n155 = call "AO AE.vi"("Mirror Modes In"=w223, "DM Value Input"=w224, "Z Comp. Input"=w225, "Action"=enum16{"READ", "WRITE"}."WRITE") -> ()  [unwired: 5 in, 3 out]
      }
      event "Capture": Value Change {
        w255 = FALSE ("element")
        n156 = event-data() -> ("CtlRef"=w263:refnum<vi>, "NewVal"=w252:variant)  [unwired: 1 in]
        n157 = call "Detectors Crl_AE.vi"() -> ("Detectors Parameters Out"=w261:T17)  [unwired: 11 in]
        n158 = Unbundle By Name(w261) -> ("PMT"=w260:bool, "Far Red (685/40 nm)"=w259:bool, "Orange (624/40 nm)"=w258:bool, "Green (525/50 nm)"=w257:bool, "Sum All"=w256:bool)
        n159 = Variant To Data(type=TRUE, Variant=w252) -> (data=w250:bool)  [unwired: 1 in, 1 out]
        n160 = Build Array(w260, w259, w258, w257, w256, w255, w255, w255) -> (w254:bool[])
        n161 = Boolean Array To Number(Boolean array=w254) -> (number=w253:u32)
        n162 = case shown="1, Default" w253 {
          tunnel: w264 -> [_ w275]
          tunnel: w263 -> [_ w274]
          tunnel: w262 -> [_ w270]
          tunnel: w250 -> [_ w269]
          frame 0 {
            w266 = FALSE ("Live")
            n163 = call "Display Message to User"() -> ()  [unwired: 10 in, 2 out]
            n164 = local write "Capture"(w266) -> ()
            n165 = local write "Live"(w266) -> ()
          }
          frame 1, Default {
            n166 = Not(x=w269) -> (.not. x?=w272:bool)
            n167 = property class="Bool (strict)"(reference=w274) -> ("Label.Text"=w271:string)  [unwired: 1 in, 2 out]
            n168 = Send Notification(notification=w272, notifier=w270) -> ()  [unwired: 1 in, 2 out]
            n169 = Select(t=w271, s=w269, f="Stop Acquisition") -> (s? t:f=w268:string)
            n170 = case shown="\"Capture\"" w271 {
              tunnel: w269 -> [_ w279 w295]
              tunnel: w268 -> [w276 w277 w294]
              tunnel: [w276 w277 w293] -> w267
              frame "False", Default {
              }
              frame "Live" {
                n171 = case shown="True" w279 {
                  tunnel: [T25."Enabled" ("Disabled") T25."Disabled and Grayed Out" ("Disabled")] -> w278
                  frame False {
                    n172 = call "Frame Counter.vi"("Action"=Counter_Action."Zero") -> ()  [unwired: 1 out]
                  }
                  frame True {
                    n173 = call "AO AE.vi"("Action"=enum16{"READ", "WRITE"}."READ") -> ("DM Value Output"=w284:dbl[][], "Z Comp. Output"=w283:T1)  [unwired: 8 in, 1 out]
                    n174 = Unbundle By Name(w283) -> ("Enable"=w282:bool)
                    n175 = call "Frame Counter.vi"("Action"=Counter_Action."Zero") -> ()  [unwired: 1 out]
                    n176 = case shown="True" w282 {
                      tunnel: w284 -> [_ w289]
                      tunnel: w283 -> [_ w288]
                      frame False {
                      }
                      frame True {
                        n177 = call "Mirror_Mode_DUAL_AE.vi"("Action"=Standard_Action."Read") -> ("Mirror Modes Out"=w291:T38)  [unwired: 14 in]
                        n178 = call "AO AE.vi"("Mirror Modes In"=w291, "DM Value Input"=w289, "Z Comp. Input"=w288, "Action"=enum16{"READ", "WRITE"}."WRITE") -> ()  [unwired: 5 in, 3 out]
                      }
                    }
                  }
                }
                n179 = property on="Capture" class="Bool (strict)"("DisabledEnum"=w278) -> ()  [unwired: 2 in, 2 out]
                n180 = property on="Exit" class="Bool"("DisabledEnum"=w278) -> ()  [unwired: 2 in, 2 out]
              }
              frame "Capture" {
                n181 = case shown="True" w295 {
                  tunnel: [T25."Enabled" ("Disabled") T25."Disabled and Grayed Out" ("Disabled")] -> w296
                  tunnel: w294 -> [w297 w310]
                  tunnel: [w297 w309] -> w293
                  frame False {
                    n182 = call "AO AE.vi"("Action"=enum16{"READ", "WRITE"}."READ") -> ("DM Value Output"=w300:dbl[][], "Z Comp. Output"=w299:T1)  [unwired: 8 in, 1 out]
                    n183 = call "Frame Counter.vi"("Action"=Counter_Action."Zero") -> ()  [unwired: 1 out]
                    n184 = Unbundle By Name(w299) -> ("Enable"=w298:bool)
                    n185 = case shown="True" w298 {
                      tunnel: w300 -> [_ w305]
                      tunnel: w299 -> [_ w304]
                      frame False {
                      }
                      frame True {
                        n186 = call "Mirror_Mode_DUAL_AE.vi"("Action"=Standard_Action."Read") -> ("Mirror Modes Out"=w307:T38)  [unwired: 14 in]
                        n187 = call "AO AE.vi"("Mirror Modes In"=w307, "DM Value Input"=w305, "Z Comp. Input"=w304, "Action"=enum16{"READ", "WRITE"}."WRITE") -> ()  [unwired: 5 in, 3 out]
                      }
                    }
                  }
                  frame True {
                    n188 = local read "Sequence"() -> (w311:T14)
                    n189 = case shown="True" w311 {
                      tunnel: w310 -> [w314 w317]
                      tunnel: [w314 w316] -> w309
                      frame False {
                      }
                      frame True {
                        n190 = call "Seq AE.vi"("Action"=enum16{"READ", "BUILD", "WRITE", "DELETE"}."READ") -> ("Array"=w315:T39)  [unwired: 8 in]
                        n191 = Array Size(array=w315) -> (size(s)=w320:i32)
                        n192 = Equal?(x=w320, y=0) -> (x = y?=w318:bool)
                        n193 = case shown="False" w318 {
                          tunnel: ["Sequence" ("f") w330] -> w316
                          tunnel: w317 -> [_ w330]
                          tunnel: w315 -> [w329 _]
                          frame False {
                            w323 = enum16{"READ", "WRITE"}."WRITE" ("Action")
                            n194 = Index Array(array=w329, index=0) -> (element=w327:T40)
                            n195 = Unbundle By Name(w327) -> ("Detectors Parameters Out"=w326:T17, "Laser Parameters Out"=w325:T18, "Image Acquisition Parameters Out"=w324:T19)
                            n196 = call "Detectors Crl_AE.vi"("Action"=w323, "Detectors Parameters In"=w326) -> ()  [unwired: 9 in, 1 out]
                            n197 = call "LASERs_ Crl_AE.vi"("Action"=w323, "Laser Parameters In"=w325) -> ()  [unwired: 9 in, 1 out]
                            n198 = call "Image Aquisition Param Ctrl_AE.vi"("Action"=w323, "Image Acquisition Parameters In"=w324) -> ()  [unwired: 9 in, 1 out]
                          }
                          frame True {
                          }
                        }
                      }
                    }
                    n199 = call "Frame Counter.vi"("Action"=Counter_Action."Zero") -> ()  [unwired: 1 out]
                  }
                }
                n200 = property on="Live" class="Bool (strict)"("DisabledEnum"=w296) -> ()  [unwired: 2 in, 2 out]
                n201 = property on="Exit" class="Bool"("DisabledEnum"=w296) -> ()  [unwired: 2 in, 2 out]
              }
            }
            n202 = Enqueue Element(queue=w275, element=w267) -> ()  [unwired: 2 in, 3 out]
          }
        }
      }
      event "Shutters": Value Change {
        n203 = event-data() -> ("CtlRef"=w334:refnum<vi>, "NewVal"=w333:variant, "OldVal"=w332:variant)  [unwired: 1 in]
        n204 = property class="Clust"(reference=w334) -> ("Label.Text"=w331:string)  [unwired: 1 in, 2 out]
        n205 = case shown="\"Image Acquisition Parameters\"" w331 {
          tunnel: w333 -> [_ w347 _ _ _]
          tunnel: w332 -> [_ w345 _ _ _]
          frame Default {
          }
          frame "Image Acquisition Parameters" {
            n206 = Variant To Data(type="Image Acquisition Parameters", Variant=w347) -> (data=w344:T19)  [unwired: 1 in, 1 out]
            n207 = Variant To Data(type=w344, Variant=w345) -> (data=w343:T19)  [unwired: 1 in, 1 out]
            n208 = Not Equal?(x=w344, y=w343) -> (x != y?=w368:T41)
            n209 = Unbundle By Name(w368) -> ("Image Dimension (um)"=w353:bool[], "Image Format"=w351:bool, "Pixel Size (nm)"=w352:bool[])
            n210 = Or Array Elements(Boolean array=w353) -> (logical OR=w357:bool)
            n211 = Or Array Elements(Boolean array=w352) -> (logical OR=w356:bool)
            n212 = Build Array(w357, w351, w356) -> (w355:bool[])
            n213 = Boolean Array To Number(Boolean array=w355) -> (number=w354:u32)
            n214 = case shown="1, 2" w354 {
              tunnel: w353 -> [_ w390 _]
              tunnel: w344 -> [w378 w383 w398]
              tunnel: [w378 w381 w396] -> w350
              tunnel: w352 -> [_ _ w395]
              tunnel: [w377 w380 w394] -> w349
              tunnel: [w376 w379 w393] -> w336
              frame 0, Default {
                n215 = Unbundle By Name(w378) -> ("Image Dimension (um)"=w377:dbl[], "Scan Mode"=w376:enum16{"XY", "XZ", "YZ", "XYZ"})
              }
              frame 1, 2 {
                # "Image Dimension or Format Change"
                n216 = Unbundle By Name(w383) -> ("Image Dimension (um)"=w389:dbl[], "Image Format"=w387:u16, "Scan Mode"=w379:enum16{"XY", "XZ", "YZ", "XYZ"})
                n217 = for {
                  tunnel: w390 -> [w392] mode=indexing
                  tunnel: w389 -> [w391] mode=indexing
                  tunnel: [w391] -> w388
                  stop <- w392 stop-if-true
                }
                n218 = To Double Precision Float(number=w387) -> (double precision float=w386:dbl)
                n219 = Build Array(w388, w388) -> (w380:dbl[])
                n220 = Divide(x=w380, y=w386) -> (x/y=w385:dbl[])
                n221 = Multiply(x=w385, y=1000.0) -> (x*y=w382:dbl[])
                n222 = Bundle By Name(cluster=w383, "Image Dimension (um)"=w380, "Pixel Size (nm)"=w382) -> (w381:T19)
              }
              frame 4 {
                # "Pixel Size Change"
                n223 = Unbundle By Name(w398) -> ("Pixel Size (nm)"=w404:dbl[], "Image Format"=w402:u16, "Scan Mode"=w393:enum16{"XY", "XZ", "YZ", "XYZ"})
                n224 = for {
                  tunnel: w395 -> [w406] mode=indexing
                  tunnel: w404 -> [w405] mode=indexing
                  tunnel: [w405] -> w403
                  stop <- w406 stop-if-true
                }
                n225 = Build Array(w403, w403) -> (w397:dbl[])
                n226 = To Double Precision Float(number=w402) -> (double precision float=w401:dbl)
                n227 = Multiply(x=w397, y=w401) -> (x*y=w400:dbl[])
                n228 = Multiply(x=w400, y=0.001) -> (x*y=w394:dbl[])
                n229 = Bundle By Name(cluster=w398, "Pixel Size (nm)"=w397, "Image Dimension (um)"=w394) -> (w396:T19)
              }
            }
            n230 = Index Array(array=w349, index=0) -> (element=w373:dbl)
            n231 = Not Equal?(x=enum16{"XY", "XZ", "YZ", "XYZ"}."YZ" ("y"), y=w336) -> (x != y?=w358:bool)
            n232 = call "Res Mirror um to Volts.vi"("Image Size (um)"=w373) -> ("Voltage (V)"=w337:dbl)
            n233 = Select(t=15780.0, s=w358, f=200.0) -> (s? t:f=w361:dbl)
            n234 = In Range and Coerce(upper limit=5.0, x=w337, lower limit=0.0) -> (coerced(x)=w339:dbl)  [unwired: 1 out]
            n235 = call "Scan Parameters Action Engine.vi"("Action"=enum16{"Read", "Write"}."Read") -> ("Scan Parameters OUT"=w340:T20)  [unwired: 14 in]
            n236 = Bundle By Name(cluster=w340, "Fast_Ax_Amp_V"=w339) -> (w338:T20)
            n237 = Bundle By Name(cluster=w350, "Fast Axis Frequency (Hz)"=w361) -> (w360:T19)
            n238 = call "Volts to I16.vi"("Voltage (V)"=w339) -> ("I16"=w372:i16)  [unwired: 13 in, 1 out]
            n239 = call "Scan Parameters Action Engine.vi"("Action"=enum16{"Read", "Write"}."Write", "Scan Parameters IN"=w338) -> ()  [unwired: 13 in, 1 out]
            n240 = call "Manual Controls Action Engine.vi"("Action"=enum16{"Read", "Write"}."Read") -> ("Manual Controls Out"=w366:T21)  [unwired: 14 in]
            n241 = Bundle By Name(cluster=w366, "Res Mirror Amp (I16)"=w372, "Res Mirror Mute"=w358) -> (w364:T21)
            n242 = call "Image Aquisition Param Ctrl_AE.vi"("Action"=enum16{"READ", "WRITE"}."WRITE", "Image Acquisition Parameters In"=w360) -> ()  [unwired: 9 in, 1 out]
            n243 = call "FPGA-7842R-Control V2.vi"("Action"=FPGA-7842R-Reference."Set Res Mirror", "Manual Controls"=w364, "Initialize"=TRUE) -> ()  [unwired: 11 in, 2 out]
            n244 = call "Manual Controls Action Engine.vi"("Action"=enum16{"Read", "Write"}."Write", "Manual Controls In"=w364) -> ()  [unwired: 13 in, 1 out]
          }
          frame "Detectors" {
            n245 = call "Detectors Crl_AE.vi"("Action"=enum16{"READ", "WRITE"}."WRITE", "Detectors Parameters In"="Detectors") -> ()  [unwired: 9 in, 1 out]
          }
          frame "Laser Controls" {
            w421 = FALSE ("element")
            n246 = Unbundle By Name("Laser Controls") -> ("STED"=w427:bool, "650 nm"=w424:bool, "590 nm"=w425:bool, "485 nm"=w426:bool, "STED Power (V)"=w418:dbl, "Manual Control"=w410:bool)
            n247 = local read "Live"() -> (w413:T14)
            n248 = call "LASERs_ Crl_AE.vi"("Action"=enum16{"READ", "WRITE"}."WRITE", "Laser Parameters In"="Laser Controls") -> ()  [unwired: 9 in, 1 out]
            n249 = Or(x=w413, y=w410) -> (x .or. y?=w412:T14)
            n250 = In Range and Coerce(upper limit=10.0, x=w418, lower limit=0.0) -> (coerced(x)=w415:dbl)  [unwired: 1 out]
            n251 = Build Array(w427, w424, w425, w426, w421, w421, w421, w421) -> (w423:bool[])
            n252 = case shown="True" w412 {
              tunnel: "Laser Controls" -> [_ w441]
              frame False {
              }
              frame True {
                n253 = call "FPGA-7842R-Control V2.vi"("Action"=FPGA-7842R-Reference."Laser Control", "Laser Controls"=w441, "Initialize"=TRUE) -> ()  [unwired: 11 in, 2 out]
              }
            }
            n254 = Boolean Array To Number(Boolean array=w423) -> (number=w422:u32)
            n255 = To Unsigned Byte Integer(number=w422) -> (unsigned 8bit integer=w420:u8)
            n256 = call "U8_To_U32.vi"("U8 IN"=w420) -> ("U32 OUT"=w419:u32)  [unwired: 13 in, 1 out]
            n257 = call "Volts to I16.vi"("Voltage (V)"=w415) -> ("I16"=w414:i16)  [unwired: 13 in, 1 out]
            n258 = case shown="False" w410 {
              tunnel: "Laser Controls" -> [w439 _]
              frame False {
                n259 = Unbundle By Name(w439) -> ("650 nm"=w436:bool, "590 nm"=w435:bool, "485 nm"=w434:bool)
                n260 = call "Detectors Crl_AE.vi"("Action"=enum16{"READ", "WRITE"}."READ") -> ("Detectors Parameters Out"=w437:T17)  [unwired: 10 in]
                n261 = Bundle By Name(cluster=w437, "Far Red (685/40 nm)"=w436, "Orange (624/40 nm)"=w435, "Green (525/50 nm)"=w434) -> (w433:T17)
                n262 = call "Detectors Crl_AE.vi"("Action"=enum16{"READ", "WRITE"}."WRITE", "Detectors Parameters In"=w433) -> ()  [unwired: 9 in, 1 out]
              }
              frame True {
              }
            }
            n263 = call "Scan Parameters Action Engine.vi"("Action"=enum16{"Read", "Write"}."Read") -> ("Scan Parameters OUT"=w430:T20)  [unwired: 14 in]
            n264 = Bundle By Name(cluster=w430, "Laser_States _U32"=w419, "775_AOM_Volt_I16"=w414) -> (w428:T20)
            n265 = call "Scan Parameters Action Engine.vi"("Action"=enum16{"Read", "Write"}."Write", "Scan Parameters IN"=w428) -> ()  [unwired: 13 in, 1 out]
          }
          frame "Shutters" {
            n266 = Unbundle By Name("Shutters") -> ("Upper Shutter"=w453:bool, "Lower Shutter"=w452:bool)
            n267 = Not(x=w453) -> (.not. x?=w444:bool)
            n268 = Not(x=w452) -> (.not. x?=w443:bool)
            n269 = call "Manual Controls Action Engine.vi"("Action"=enum16{"Read", "Write"}."Read") -> ("Manual Controls Out"=w448:T21)  [unwired: 14 in]
            n270 = Bundle By Name(cluster=w448, "Upper Shutter"=w444, "Lower Shutter"=w443) -> (w445:T21)
            n271 = call "Manual Controls Action Engine.vi"("Action"=enum16{"Read", "Write"}."Write", "Manual Controls In"=w445) -> ()  [unwired: 13 in, 1 out]
            n272 = call "FPGA-7842R-Control V2.vi"("Action"=FPGA-7842R-Reference."Shutter Control", "Manual Controls"=w445, "Initialize"=TRUE) -> ()  [unwired: 11 in, 2 out]
          }
        }
      }
      event Value Change {
        # "For P541 - Sample Z - Converting from Step in µm to I16 is as follows. We have (Step µw)*(10 V / 100 µm)*(32768 I16 / 10 V) = (Step µm)*(32768 I16 / 100 µm) = (Step µm)*(327.68 I16/µm)"
        n273 = event-data() -> ("CtlRef"=w467:refnum<vi>, "OldVal"=w465:variant, "NewVal"=w466:variant)  [unwired: 1 in]
        n274 = local write "Abort AllStage"(FALSE ("Abort AllStage")) -> ()
        n275 = property class="Clust"(reference=w467) -> ("Label.Text"=w464:string)  [unwired: 1 in, 2 out]
        n276 = case shown="\"Sample Stage XY - M686\"" w464 {
          tunnel: w466 -> [_ w490 w531 w558 w621 w662 w691 w730]
          tunnel: w465 -> [_ w489 w530 w557 w622 w663 w692 w731]
          tunnel: ["" "N664" "ASI" "P612" "P612" "P841" "M227" "M686"] -> w463
          tunnel: [dbl[] [0.0] w481 w523 w546 dbl[] [0.0] w651 w684 w720] -> w462
          tunnel: [bool[] [FALSE] w479 w517 w547 bool[] [FALSE] bool[] [TRUE] w685 w719] -> w461
          tunnel: [enum16{"MOVE", "MVR"}."MVR" ("MOVE/MVR") w478 w520 w549 enum16{"MOVE", "MVR"}."MVR" ("MOVE/MVR") w654 w677 w722] -> w460
          tunnel: [0.0 ("Step Size (um)") 0.5 ("Step Size (um)") w522 0.0 ("Velocity") 0.0 ("Velocity") 10000.0 ("Velocity") 0.0 ("Velocity") 0.0 ("Velocity")] -> w456
          tunnel: [StageStates."MVR" ("Action") w476 w521 w550 StageStates."POSITION" ("Action") w655 w681 w723] -> w454
          frame Default {
          }
          frame "Upper Objective Z - N664" {
            n277 = call "N664_Ctrl_Index.vi"("OldVal"=w489, "NewVal"=w490) -> ("Control Ref OUT"=w488:refnum<vi>, "N664 Out"=w486:T6)  [unwired: 12 in]
            n278 = property class="Ctl"(reference=w488) -> ("Label.Text"=w487:string)  [unwired: 1 in, 2 out]
            n279 = Unbundle By Name(w486) -> ("Step Size (um)"=w485:dbl, "Position (mm)"=w484:dbl)
            n280 = case shown="\"Home\"" w487 {
              tunnel: w485 -> [_ w495 w498 _ _ _]
              tunnel: [0.0 ("Step Size (um)") w494 w498 w503 w505 w510] -> w482
              tunnel: w484 -> [_ _ _ w503 w505 _]
              tunnel: [enum16{"MOVE", "MVR"}."MVR" ("MOVE/MVR") enum16{"MOVE", "MVR"}."MVR" ("MOVE/MVR") enum16{"MOVE", "MVR"}."MVR" ("MOVE/MVR") enum16{"MOVE", "MVR"}."MOVE" ("MOVE/MVR") enum16{"MOVE", "MVR"}."MOVE" ("MOVE/MVR") enum16{"MOVE", "MVR"}."MOVE" ("MOVE/MVR")] -> w478
              tunnel: [StageStates."MVR" ("Action") StageStates."MVR" ("Action") StageStates."MVR" ("Action") StageStates."MOVE" ("Action") StageStates."MOVE" ("Action") StageStates."MOVE" ("Action")] -> w476
              frame Default {
              }
              frame "Up N664" {
                n281 = Negate(x=w495) -> (-x=w494:dbl)
              }
              frame "Down N664" {
              }
              frame "Position (mm)" {
              }
              frame "Save" {
                n282 = Build Array(w505) -> (w504:dbl[])
                n283 = call "Stage_position_ae.vi"("Position In"=w504, "StageID"="N664", "Enum"=enum16{"WRITE", "READ", "HOME", "SAVE HOME"}."SAVE HOME") -> ()  [unwired: 7 in, 2 out]
              }
              frame "Home" {
                n284 = call "Stage_position_ae.vi"("StageID"="N664", "Enum"=enum16{"WRITE", "READ", "HOME", "SAVE HOME"}."HOME") -> ("Position Out"=w512:dbl[])  [unwired: 8 in, 1 out]
                n285 = Index Array(array=w512, index=0) -> (element=w510:dbl)
              }
            }
            n286 = Build Array(w482) -> (w481:dbl[])
            n287 = Build Array(TRUE) -> (w479:bool[])
          }
          frame "Cavity Translation Z - ASI" {
            n288 = call "ASI_Ctrl_Index.vi"("NewVal"=w531, "OldVal"=w530) -> ("ASI out"=w527:T7, "Control Ref OUT"=w529:refnum<vi>)  [unwired: 8 in]
            n289 = property class="Ctl"(reference=w529) -> ("Label.Text"=w528:string)  [unwired: 1 in, 2 out]
            n290 = Unbundle By Name(w527) -> ("Step Size (um)"=w526:dbl, "Z (um)"=w525:dbl, "Velocity"=w522:dbl)
            n291 = case shown="\"Z (um)\"" w528 {
              tunnel: w526 -> [_ w537 w540 _]
              tunnel: w525 -> [_ _ _ w544]
              tunnel: [0.0 ("Z (um)") w537 w541 w544] -> w524
              tunnel: [StageStates."MVR" ("Action") StageStates."MVR" ("Action") StageStates."MVR" ("Action") StageStates."MOVE" ("Action")] -> w521
              tunnel: [enum16{"MOVE", "MVR"}."MVR" ("MOVE/MVR") enum16{"MOVE", "MVR"}."MVR" ("MOVE/MVR") enum16{"MOVE", "MVR"}."MVR" ("MOVE/MVR") enum16{"MOVE", "MVR"}."MOVE" ("MOVE/MVR")] -> w520
              frame Default {
              }
              frame "Up ASI" {
              }
              frame "Down ASI" {
                n292 = Negate(x=w540) -> (-x=w541:dbl)
              }
              frame "Z (um)" {
              }
            }
            n293 = Build Array(w524) -> (w523:dbl[])
            n294 = Build Array(TRUE) -> (w517:bool[])
          }
          frame "Bottom Objective XY - P612" {
            n295 = call "P612_Ctrl_Index.vi"("OldVal"=w557, "NewVal"=w558) -> ("Control out"=w556:refnum<vi>, "P612 out"=w554:T10)  [unwired: 12 in]
            n296 = property class="Ctl"(reference=w556) -> ("Label.Text"=w555:string)  [unwired: 1 in, 2 out]
            n297 = Unbundle By Name(w554) -> ("Step Size (um)"=w553:dbl, "X"=w552:dbl, "Y"=w551:dbl)
            n298 = case shown="\"Up Button\"" w555 {
              tunnel: w553 -> [_ _ w569 w576 w580 w587 _]
              tunnel: w552 -> [_ _ _ _ _ _ w594]
              tunnel: w551 -> [_ _ _ _ _ _ w593]
              tunnel: [StageStates."MVR" ("Action") StageStates."HOME" ("Action") StageStates."MVR" ("Action") StageStates."MVR" ("Action") StageStates."MVR" ("Action") StageStates."MVR" ("Action") StageStates."MOVE" ("Action")] -> w550
              tunnel: [enum16{"MOVE", "MVR"}."MVR" ("MOVE/MVR") enum16{"MOVE", "MVR"}."MVR" ("MOVE/MVR") enum16{"MOVE", "MVR"}."MVR" ("MOVE/MVR") enum16{"MOVE", "MVR"}."MVR" ("MOVE/MVR") enum16{"MOVE", "MVR"}."MVR" ("MOVE/MVR") enum16{"MOVE", "MVR"}."MVR" ("MOVE/MVR") enum16{"MOVE", "MVR"}."MOVE" ("MOVE/MVR")] -> w549
              tunnel: [bool[] [FALSE] bool[] [TRUE, TRUE] bool[] [TRUE, FALSE] bool[] [TRUE, FALSE] bool[] [FALSE, TRUE] bool[] [FALSE, TRUE] bool[] [TRUE, TRUE]] -> w547
              tunnel: [dbl[] [0.0] dbl[] [0.0, 0.0] w568 w575 w582 w589 w595] -> w546
              frame Default {
              }
              frame "Home Button" {
              }
              frame "Up Button" {
                n299 = Build Array(w569, 0.0 ("element")) -> (w568:dbl[])
              }
              frame "Down Button" {
                n300 = Negate(x=w576) -> (-x=w573:dbl)
                n301 = Build Array(w573, 0.0 ("element")) -> (w575:dbl[])
              }
              frame "Left Button" {
                n302 = Build Array(0.0 ("element"), w580) -> (w582:dbl[])
              }
              frame "Right Button" {
                n303 = Negate(x=w587) -> (-x=w586:dbl)
                n304 = Build Array(0.0 ("element"), w586) -> (w589:dbl[])
              }
              frame "X", "Y" {
                n305 = Build Array(w594, w593) -> (w595:dbl[])
              }
            }
          }
          frame "Sample Z - P541" {
            w600 = 327.68 ("y")
            n306 = call "P541_Ctrl_Index.vi"("OldVal"=w622, "NewVal"=w621) -> ("Control out"=w620:refnum<vi>, "P541 Out"=w619:T16)  [unwired: 12 in]
            n307 = Unbundle By Name(w619) -> ("Z Position"=w599:dbl, "Step Size (um)"=w618:dbl)
            n308 = property class="Ctl"(reference=w620) -> ("Label.Text"=w617:string)  [unwired: 1 in, 2 out]
            n309 = call "Manual Controls Action Engine.vi"("Action"=enum16{"Read", "Write"}."Read") -> ("Manual Controls Out"=w608:T21)  [unwired: 14 in]
            n310 = Unbundle By Name(w608) -> ("Z Axis Voltage (I16)"=w611:i16)
            n311 = Multiply(x=w599, y=w600) -> (x*y=w614:dbl)
            n312 = Multiply(x=w618, y=w600) -> (x*y=w616:dbl)
            n313 = Round To Nearest(number=w614) -> (nearest integer value=w603:dbl)
            n314 = Round To Nearest(number=w616) -> (nearest integer value=w602:dbl)
            n315 = To Word Integer(number=w603) -> (16bit integer=w613:i16)
            n316 = To Word Integer(number=w602) -> (16bit integer=w615:i16)
            n317 = case shown="\"Home\"" w617 {
              tunnel: w615 -> [_ w629 w633 _ _ _]
              tunnel: w613 -> [_ _ _ w635 _ _]
              tunnel: w611 -> [w628 w631 w634 _ w640 _]
              tunnel: [w628 w630 w632 w635 w640 w646] -> w607
              tunnel: w600 -> [_ _ _ _ _ w645]
              tunnel: w599 -> [_ _ _ _ w639 _]
              frame Default {
              }
              frame "Step Down" {
                n318 = Subtract(x=w631, y=w629) -> (x-y=w630:i16)
              }
              frame "Step Up" {
                n319 = Add(x=w634, y=w633) -> (x+y=w632:i16)
              }
              frame "Z Position" {
              }
              frame "Save" {
                n320 = Build Array(w639) -> (w638:dbl[])
                n321 = call "Stage_position_ae.vi"("Position In"=w638, "StageID"="P541", "Enum"=enum16{"WRITE", "READ", "HOME", "SAVE HOME"}."SAVE HOME") -> ()  [unwired: 7 in, 2 out]
              }
              frame "Home" {
                n322 = call "Stage_position_ae.vi"("StageID"="P541", "Enum"=enum16{"WRITE", "READ", "HOME", "SAVE HOME"}."HOME") -> ("Position Out"=w643:dbl[])  [unwired: 8 in, 1 out]
                n323 = Index Array(array=w643, index=0) -> (element=w641:dbl)
                n324 = Multiply(x=w641, y=w645) -> (x*y=w647:dbl)
                n325 = Round To Nearest(number=w647) -> (nearest integer value=w648:dbl)
                n326 = To Word Integer(number=w648) -> (16bit integer=w646:i16)
              }
            }
            n327 = Bundle By Name(cluster=w608, "Z Axis Voltage (I16)"=w607) -> (w610:T21)
            n328 = call "Manual Controls Action Engine.vi"("Action"=enum16{"Read", "Write"}."Write", "Manual Controls In"=w610) -> ("Manual Controls Out"=w604:T21)  [unwired: 13 in]
            n329 = call "FPGA-7842R-Control V2.vi"("Action"=FPGA-7842R-Reference."Stage Control", "Manual Controls"=w604, "Initialize"=TRUE) -> ()  [unwired: 11 in, 2 out]
          }
          frame "Phase Comp Mirror - P841" {
            n330 = call "P841_Ctrl_Index.vi"("OldVal"=w663, "NewVal"=w662) -> ("Control out"=w660:refnum<vi>, "P841 Out"=w658:T8)  [unwired: 12 in]
            n331 = property class="Ctl"(reference=w660) -> ("Label.Text"=w659:string)  [unwired: 1 in, 2 out]
            n332 = Unbundle By Name(w658) -> ("Position (µm)"=w657:dbl, "Step Size (µm)"=w656:dbl)
            n333 = case shown="Default" w659 {
              tunnel: w657 -> [_ _ _ w676]
              tunnel: w656 -> [_ w669 w673 _]
              tunnel: [0.0 ("Position (µm)") w669 w672 w676] -> w652
              tunnel: [StageStates."MVR" ("Action") StageStates."MVR" ("Action") StageStates."MVR" ("Action") StageStates."MOVE" ("Action")] -> w655
              tunnel: [enum16{"MOVE", "MVR"}."MVR" ("MOVE/MVR") enum16{"MOVE", "MVR"}."MVR" ("MOVE/MVR") enum16{"MOVE", "MVR"}."MVR" ("MOVE/MVR") enum16{"MOVE", "MVR"}."MOVE" ("MOVE/MVR")] -> w654
              frame Default {
              }
              frame "Up P841" {
              }
              frame "Down P841" {
                n334 = Negate(x=w673) -> (-x=w672:dbl)
              }
              frame "Position (µm)" {
              }
            }
            n335 = Build Array(w652) -> (w651:dbl[])
          }
          frame "Sample Z Coarse - M227" {
            n336 = call "M227_Ctrl_Index.vi"("OldVal"=w692, "NewVal"=w691) -> ("Control Ref OUT"=w690:refnum<vi>, "M227 Out"=w688:T12)  [unwired: 12 in]
            n337 = property class="Ctl"(reference=w690) -> ("Label.Text"=w689:string)  [unwired: 1 in, 2 out]
            n338 = Unbundle By Name(w688) -> ("Step Size (mm)"=w687:dbl, "MM 1"=w680:dbl, "MM 2"=w679:dbl, "MM 3"=w678:dbl)
            n339 = case shown="\"MM 1\"" w689 {
              tunnel: w687 -> [_ _ _ _ w711 w716]
              tunnel: [bool[] [FALSE, FALSE, FALSE] bool[] [TRUE, TRUE, TRUE] bool[] [TRUE, TRUE, TRUE] bool[] [TRUE, TRUE, TRUE] bool[] [TRUE, TRUE, TRUE] bool[] [TRUE, TRUE, TRUE]] -> w685
              tunnel: [0.0 ("Step Size (mm)") w698 w702 w706 w711 w715] -> w682
              tunnel: [StageStates."POSITION" ("Action") StageStates."MOVE" ("Action") StageStates."MOVE" ("Action") StageStates."MOVE" ("Action") StageStates."MVR" ("Action") StageStates."MVR" ("Action")] -> w681
              tunnel: w680 -> [_ w698 _ _ _ _]
              tunnel: w679 -> [_ _ w702 _ _ _]
              tunnel: w678 -> [_ _ _ w706 _ _]
              tunnel: [enum16{"MOVE", "MVR"}."MVR" ("MOVE/MVR") enum16{"MOVE", "MVR"}."MOVE" ("MOVE/MVR") enum16{"MOVE", "MVR"}."MOVE" ("MOVE/MVR") enum16{"MOVE", "MVR"}."MOVE" ("MOVE/MVR") enum16{"MOVE", "MVR"}."MVR" ("MOVE/MVR") enum16{"MOVE", "MVR"}."MVR" ("MOVE/MVR")] -> w677
              frame Default {
              }
              frame "MM 1" {
              }
              frame "MM 2" {
              }
              frame "MM 3" {
              }
              frame "Up M227" {
              }
              frame "Down M227" {
                n340 = Negate(x=w716) -> (-x=w715:dbl)
              }
            }
            n341 = Build Array(w682, w682, w682) -> (w684:dbl[])
          }
          frame "Sample Stage XY - M686" {
            n342 = call "M686_Ctrl_Index.vi"("NewVal"=w730, "OldVal"=w731) -> ("M686 - out"=w728:T9, "Control out"=w729:refnum<vi>)  [unwired: 8 in]
            n343 = Unbundle By Name(w728) -> ("Step Size (um)"=w727:dbl, "X"=w726:dbl, "Y"=w725:dbl)
            n344 = property class="Ctl"(reference=w729) -> ("Label.Text"=w718:string)  [unwired: 1 in, 2 out]
            n345 = case shown="\"Left Button\"" w718 {
              tunnel: w727 -> [_ _ w743 w748 w756 w761 _]
              tunnel: w726 -> [_ _ _ _ _ _ w768]
              tunnel: w725 -> [_ _ _ _ _ _ w767]
              tunnel: [StageStates."POSITION" ("Action") StageStates."MOVE" ("Action") StageStates."MVR" ("Action") StageStates."MVR" ("Action") StageStates."MVR" ("Action") StageStates."MVR" ("Action") StageStates."MOVE" ("Action")] -> w723
              tunnel: [enum16{"MOVE", "MVR"}."MVR" ("MOVE/MVR") enum16{"MOVE", "MVR"}."MOVE" ("MOVE/MVR") enum16{"MOVE", "MVR"}."MVR" ("MOVE/MVR") enum16{"MOVE", "MVR"}."MVR" ("MOVE/MVR") enum16{"MOVE", "MVR"}."MVR" ("MOVE/MVR") enum16{"MOVE", "MVR"}."MVR" ("MOVE/MVR") enum16{"MOVE", "MVR"}."MOVE" ("MOVE/MVR")] -> w722
              tunnel: [w733 dbl[] [12.5, 12.5] w741 w749 w757 w763 w769] -> w720
              tunnel: [bool[] [FALSE, FALSE] bool[] [TRUE, TRUE] bool[] [TRUE, TRUE] bool[] [TRUE, TRUE] bool[] [TRUE, TRUE] bool[] [TRUE, TRUE] bool[] [TRUE, TRUE]] -> w719
              frame Default {
                w734 = 0.0 ("Step Size (mm)")
                n346 = Build Array(w734, w734) -> (w733:dbl[])
              }
              frame "Home Button" {
              }
              frame "Right Button" {
                n347 = Build Array(w743, 0.0 ("element")) -> (w741:dbl[])
              }
              frame "Left Button" {
                n348 = Negate(x=w748) -> (-x=w747:dbl)
                n349 = Build Array(w747, 0.0 ("element")) -> (w749:dbl[])
              }
              frame "Up Button" {
                n350 = Negate(x=w756) -> (-x=w755:dbl)
                n351 = Build Array(0.0 ("element"), w755) -> (w757:dbl[])
              }
              frame "Down Button" {
                n352 = Build Array(0.0 ("element"), w761) -> (w763:dbl[])
              }
              frame "X", "Y" {
                n353 = Build Array(w768, w767) -> (w769:dbl[])
              }
            }
          }
        }
        n354 = case shown="Default" w464 {
          frame Default {
          }
          frame "Upper Objective Z - N664" {
            n355 = while {
              i -> [w778]
              stop <- w774 stop-if-true
              n356 = call "Stage_position_ae.vi"("StageID"="N664", "Enum"=enum16{"WRITE", "READ", "HOME", "SAVE HOME"}."READ") -> ("Status Out"=w775:bool, "Position Out"=w785:dbl[])  [unwired: 8 in]
              n357 = Greater?(x=w778, y=200) -> (0:w777:bool)
              n358 = And(x=w775, y=w777) -> (x .and. y?=w774:bool)
              n359 = Wait (ms)(milliseconds to wait=u32 1) -> ()  [unwired: 1 out]
              n360 = Index Array(array=w785, index=0) -> (element=w784:dbl)
              n361 = Select(t=u32 16777215, s=w774, f=u32 6618880) -> (s? t:f=w779:u32)
              n362 = property on="Position (mm)" class="DigNum (strict)"("Value"=w784, "NumText.BG Color"=w779) -> ()  [unwired: 2 in, 2 out]
            }
          }
          frame "Cavity Translation Z - ASI" {
            n363 = while {
              shift-right: [w792] -> _
              shift-left: TRUE ("Status Out") -> [w797]
              stop <- w796 stop-if-true
              n364 = call "Stage_position_ae.vi"("StageID"="ASI", "Enum"=enum16{"WRITE", "READ", "HOME", "SAVE HOME"}."READ") -> ("Status Out"=w792:bool, "Position Out"=w800:dbl[])  [unwired: 8 in]
              n365 = Greater?(x=w792, y=w797) -> (0:w796:bool)
              n366 = Wait (ms)(milliseconds to wait=u32 1) -> ()  [unwired: 1 out]
              n367 = Index Array(array=w800, index=0) -> (element=w790:dbl)
              n368 = Divide(x=w790, y=10.0) -> (x/y=w791:dbl)
              n369 = Select(t=u32 16777215, s=w792, f=u32 6618880) -> (s? t:f=w793:u32)
              n370 = property on="Z (um)" class="DigNum (strict)"("Value"=w791, "NumText.BG Color"=w793) -> ()  [unwired: 2 in, 2 out]
            }
          }
        }
        n371 = control-ref of="Abort AllStage"() -> (w455:refnum<vi>)
        n372 = call "AllStage_Limits_Array.vi"("Step(um)/Position(units)"=w462, "Axis"=w461, "Stage ID"=w463, "MOVE/MVR"=w460) -> ("Positions"=w458:dbl[], "Boolean Array"=w457:bool[], "Stage ID"=w459:string)  [unwired: 4 in, 1 out]
        n373 = call "AE_AllStages_Action V2.vi"("Velocity"=w456, "Abort"=w455, "Positions"=w458, "Axis"=w457, "Stage ID"=w459, "Action"=w454) -> ()  [unwired: 3 in, 3 out]
      }
      event "Stages": Value Change {
        n374 = event-data() -> ("NewVal"=w814:T11)  [unwired: 1 in, 2 out]
        n375 = Unbundle By Name(w814) -> ("M686"=w802:bool, "P841"=w812:bool, "ASI"=w810:bool, "N664"=w808:bool, "P612"=w806:bool, "M227"=w804:bool)
        n376 = call "All_Stages_Aloha.vi"("Aloha"=w802, "Stage ID"="M686") -> ()  [unwired: 9 in, 1 out]
        n377 = call "All_Stages_Aloha.vi"("Aloha"=w812, "Stage ID"="P841") -> ()  [unwired: 9 in, 1 out]
        n378 = call "All_Stages_Aloha.vi"("Aloha"=w810, "Stage ID"="ASI") -> ()  [unwired: 9 in, 1 out]
        n379 = call "All_Stages_Aloha.vi"("Aloha"=w808, "Stage ID"="N664") -> ()  [unwired: 9 in, 1 out]
        n380 = call "All_Stages_Aloha.vi"("Aloha"=w806, "Stage ID"="P612") -> ()  [unwired: 9 in, 1 out]
        n381 = call "All_Stages_Aloha.vi"("Aloha"=w804, "Stage ID"="M227") -> ()  [unwired: 9 in, 1 out]
      }
      event Value Change {
        n382 = event-data() -> ("CtlRef"=w818:refnum<vi>, "NewVal"=w815:T14)  [unwired: 1 in, 1 out]
        n383 = property class="Bool (strict)"(reference=w818) -> ("Label.Text"=w817:string)  [unwired: 1 in, 2 out]
        n384 = case shown="\"SLM\", Default" w817 {
          tunnel: w815 -> [w819 w833 w847 w851 w865 w878 w895]
          frame "SLM", Default {
            n385 = case shown="True" w819 {
              frame False {
                n386 = To Variant(anything=TRUE) -> (Variant=w825:variant)
                n387 = call "SLM AE.vi"("Action"=enum16{"READ", "WRITE"}."READ") -> ("SLM Ref Out"=w826:refnum<vi>)  [unwired: 10 in]
                n388 = invoke class="VI" method="Ctrl Val.Set"(reference=w826, "Control Name"="Exit", "Value"=w825) -> (reference out=w822:refnum<vi>, error out=w821:errorcluster)  [unwired: 2 in, 3 out]
                n389 = invoke on="Hamamatsu LCOS" class="SubPnl" method="Remove VI"(error in=w821) -> (error out=w820:errorcluster)  [unwired: 2 in, 2 out]
                n390 = Close Reference(reference=w822, error in (no error)=w820) -> ()  [unwired: 1 out]
              }
              frame True {
                n391 = Open VI Reference(vi path=path "C:/Users/ED STED/Documents/Test Control Software/Host VIs/SLM_V3_DL/SLM Control.vi") -> (vi reference=w831:refnum<vi>)  [unwired: 5 in, 1 out]
                n392 = invoke class="VI" method="Run VI"(reference=w831, "Wait until done"=FALSE ("Wait Until Done")) -> (reference out=w828:refnum<vi>)  [unwired: 3 in, 4 out]
                n393 = invoke on="Hamamatsu LCOS" class="SubPanel" method="Insert VI"("VI Ref"=w828) -> ()  [unwired: 3 in, 4 out]
                n394 = call "SLM AE.vi"("Action"=enum16{"READ", "WRITE"}."WRITE", "SLM Ref In"=w828) -> ()  [unwired: 9 in, 1 out]
              }
            }
          }
          frame "DM" {
            n395 = case shown="True" w833 {
              frame False {
                n396 = call "DM_Ref_AE.vi"("Action"=enum16{"READ", "WRITE"}."READ") -> ("DM Ref Out"=w840:refnum<vi>)  [unwired: 10 in]
                n397 = To Variant(anything=TRUE) -> (Variant=w839:variant)
                n398 = invoke class="VI" method="Ctrl Val.Set"(reference=w840, "Control Name"="Exit", "Value"=w839) -> (reference out=w836:refnum<vi>, error out=w835:errorcluster)  [unwired: 2 in, 3 out]
                n399 = invoke on="BM Multi" class="SubPnl" method="Remove VI"(error in=w835) -> (error out=w834:errorcluster)  [unwired: 2 in, 2 out]
                n400 = Close Reference(reference=w836, error in (no error)=w834) -> ()  [unwired: 1 out]
              }
              frame True {
                n401 = Open VI Reference(vi path=path "C:/Users/ED STED/Documents/Test Control Software/Host VIs/DM_Dual_V2/Dual_DM_Control_Main_V6.vi") -> (vi reference=w845:refnum<vi>)  [unwired: 5 in, 1 out]
                n402 = invoke class="VI" method="Run VI"(reference=w845, "Wait until done"=FALSE ("Wait Until Done")) -> (reference out=w842:refnum<vi>)  [unwired: 3 in, 4 out]
                n403 = invoke on="BM Multi" class="SubPanel" method="Insert VI"("VI Ref"=w842) -> ()  [unwired: 3 in, 4 out]
                n404 = call "DM_Ref_AE.vi"("Action"=enum16{"READ", "WRITE"}."WRITE", "DM Ref In"=w842) -> ()  [unwired: 9 in, 1 out]
              }
            }
          }
          frame "Sequence" {
            n405 = case shown="False" w847 {
              tunnel: [T25."Disabled and Grayed Out" ("Disabled") T25."Enabled" ("Disabled")] -> w848
              frame False {
              }
              frame True {
              }
            }
            n406 = property on="Sequence Cluster" class="Clust"("DisabledEnum"=w848) -> ()  [unwired: 2 in, 2 out]
          }
          frame "Timing" {
            n407 = case shown="True" w851 {
              frame False {
                n408 = To Variant(anything=TRUE) -> (Variant=w856:variant)
                n409 = call "GateDelay AE.vi"("Action"=enum16{"READ", "WRITE"}."READ") -> ("Gate Delay Ref Out"=w857:refnum<vi>)  [unwired: 10 in]
                n410 = invoke class="VI" method="Ctrl Val.Set"(reference=w857, "Control Name"="Exit", "Value"=w856) -> (reference out=w852:refnum<vi>, error out=w853:errorcluster)  [unwired: 2 in, 3 out]
                n411 = invoke on="Timing" class="SubPnl" method="Remove VI"(error in=w853) -> (error out=w859:errorcluster)  [unwired: 2 in, 2 out]
                n412 = Close Reference(reference=w852, error in (no error)=w859) -> ()  [unwired: 1 out]
              }
              frame True {
                n413 = Open VI Reference(vi path=path "C:/Users/ED STED/Documents/Test Control Software/Host VIs/Time Delay/GateDelay_Control_V3.vi") -> (vi reference=w862:refnum<vi>)  [unwired: 5 in, 1 out]
                n414 = invoke class="VI" method="Run VI"(reference=w862, "Wait until done"=FALSE ("Wait Until Done")) -> (reference out=w861:refnum<vi>)  [unwired: 3 in, 4 out]
                n415 = invoke on="Timing" class="SubPanel" method="Insert VI"("VI Ref"=w861) -> ()  [unwired: 3 in, 4 out]
                n416 = call "GateDelay AE.vi"("Action"=enum16{"READ", "WRITE"}."WRITE", "Gate Delay Ref In"=w861) -> ()  [unwired: 9 in, 1 out]
              }
            }
          }
          frame "Camera" {
            n417 = case shown="False" w865 {
              frame False {
                n418 = To Variant(anything=TRUE) -> (Variant=w866:variant)
                n419 = call "Camera_Ref_HX.vi"("Action"=enum16{"READ", "WRITE"}."READ") -> ("Alignment Ref Out"=w870:refnum<vi>)  [unwired: 10 in]
                n420 = invoke class="VI" method="Ctrl Val.Set"(reference=w870, "Control Name"="Exit", "Value"=w866) -> (reference out=w869:refnum<vi>)  [unwired: 2 in, 4 out]
                n421 = invoke on="Tool Box" class="SubPnl" method="Remove VI"() -> (error out=w871:errorcluster)  [unwired: 3 in, 2 out]
                n422 = Close Reference(reference=w869, error in (no error)=w871) -> ()  [unwired: 1 out]
              }
              frame True {
                n423 = Open VI Reference(vi path=path "C:/Users/ED STED/Documents/Test Control Software/Host VIs/Camera/uEye_Control_V1.vi") -> (vi reference=w875:refnum<vi>)  [unwired: 5 in, 1 out]
                n424 = invoke class="VI" method="Run VI"(reference=w875, "Wait until done"=FALSE ("Wait Until Done")) -> (reference out=w874:refnum<vi>)  [unwired: 3 in, 4 out]
                n425 = invoke on="Tool Box" class="SubPnl" method="Insert VI"("VI Ref"=w874) -> ()  [unwired: 3 in, 4 out]
                n426 = call "Camera_Ref_HX.vi"("Action"=enum16{"READ", "WRITE"}."WRITE", "Alignment Ref In"=w874) -> ()  [unwired: 9 in, 1 out]
              }
            }
          }
          frame "Focus Lock" {
            n427 = case shown="True" w878 {
              frame False {
                n428 = call "Lock Control AE.vi"("Action"=Standard_Action_for_Focus_Lock."Read") -> ("Lock Control  out"=w881:T42)  [unwired: 1 in]
                n429 = Bundle By Name(cluster=w881, "EXIT"=TRUE) -> (w879:T42)
                n430 = call "FocusLock_Ref_HX.vi"("Action"=enum16{"READ", "WRITE"}."READ") -> ("FocusLock Ref Out"=w887:refnum<vi>)  [unwired: 10 in]
                n431 = To Variant(anything=w879) -> (Variant=w885:variant)
                n432 = invoke class="VI" method="Ctrl Val.Set"(reference=w887, "Control Name"="Lock Control", "Value"=w885) -> (reference out=w886:refnum<vi>, error out=w884:errorcluster)  [unwired: 2 in, 3 out]
                n433 = invoke on="Focus Lock\nFocus Lock Panel" class="SubPnl" method="Remove VI"(error in=w884) -> (error out=w888:errorcluster)  [unwired: 2 in, 2 out]
                n434 = Close Reference(reference=w886, error in (no error)=w888) -> ()  [unwired: 1 out]
              }
              frame True {
                n435 = Open VI Reference(vi path=path "C:/Users/ED STED/Documents/Test Control Software/Host VIs/Focus Lock/FocusLock Control v3.vi") -> (vi reference=w892:refnum<vi>)  [unwired: 5 in, 1 out]
                n436 = invoke class="VI" method="Run VI"(reference=w892, "Wait until done"=FALSE ("Wait Until Done")) -> (reference out=w891:refnum<vi>)  [unwired: 3 in, 4 out]
                n437 = invoke on="Focus Lock\nFocus Lock Panel" class="SubPnl" method="Insert VI"("VI Ref"=w891) -> ()  [unwired: 3 in, 4 out]
                n438 = call "FocusLock_Ref_HX.vi"("Action"=enum16{"READ", "WRITE"}."WRITE", "FocusLock Ref In"=w891) -> ()  [unwired: 9 in, 1 out]
              }
            }
          }
          frame "Stage Monitor" {
            n439 = case shown="True" w895 {
              frame False {
                n440 = call "StageMonitor_Ref_HX.vi"("Action"=enum16{"READ", "WRITE"}."READ") -> ("StageMonitor Ref Out"=w898:refnum<vi>)  [unwired: 10 in]
                n441 = To Variant(anything=TRUE) -> (Variant=w901:variant)
                n442 = invoke class="VI" method="Ctrl Val.Set"(reference=w898, "Control Name"="Exit", "Value"=w901) -> (reference out=w902:refnum<vi>, error out=w900:errorcluster)  [unwired: 2 in, 3 out]
                n443 = invoke on="Tool Box 2" class="SubPnl" method="Remove VI"(error in=w900) -> (error out=w903:errorcluster)  [unwired: 2 in, 2 out]
                n444 = Close Reference(reference=w902, error in (no error)=w903) -> ()  [unwired: 1 out]
              }
              frame True {
                n445 = Open VI Reference(vi path=path "C:/Users/ED STED/Documents/Test Control Software/Host VIs/Stages/Stage Monitor/Stage Monitor.vi") -> (vi reference=w906:refnum<vi>)  [unwired: 5 in, 1 out]
                n446 = invoke class="VI" method="Run VI"(reference=w906, "Wait until done"=FALSE ("Wait Until Done")) -> (reference out=w905:refnum<vi>)  [unwired: 3 in, 4 out]
                n447 = invoke on="Tool Box 2" class="SubPnl" method="Insert VI"("VI Ref"=w905) -> ()  [unwired: 3 in, 4 out]
                n448 = call "StageMonitor_Ref_HX.vi"("Action"=enum16{"READ", "WRITE"}."WRITE", "StageMonitor Ref In"=w905) -> ()  [unwired: 9 in, 1 out]
              }
            }
          }
        }
      }
      event Value Change {
        n449 = event-data() -> ("CtlRef"=w914:refnum<vi>, "OldVal"=w912:variant, "NewVal"=w911:variant)  [unwired: 1 in]
        n450 = property class="Clust"(reference=w914) -> ("Label.Text"=w913:string)  [unwired: 1 in, 2 out]
        n451 = call "Graph Ref AE.vi"("Action"=enum16{"READ", "WRITE"}."READ") -> ("Graph Ref Out"=w909:refnum<vi>[])  [unwired: 10 in]
        n452 = case shown="\"Graph Tools\"" w913 {
          tunnel: w912 -> [_ w921 w977]
          tunnel: w911 -> [_ w922 w976]
          tunnel: w909 -> [_ w916 w969]
          frame Default {
          }
          frame "Display Controls" {
            n453 = call "Display_Controls_Ctrl_Index.vi"("OldVal"=w921, "NewVal"=w922) -> ("Control Ref OUT"=w920:refnum<vi>, "Display Controls Out"=w918:T3)  [unwired: 12 in]
            n454 = property class="Ctl"(reference=w920) -> ("Label.Text"=w919:string)  [unwired: 1 in, 2 out]
            n455 = Unbundle By Name(w918) -> ("Single Screen"=w917:bool)
            n456 = case shown="\"Single Screen\", Default" w919 {
              tunnel: w917 -> [w930 _ _]
              tunnel: w916 -> [_ w955 w962]
              frame "Single Screen", Default {
                n457 = property class="App"() -> ("Disp.AllMonitors"=w929:T43)  [unwired: 2 in, 2 out]
                n458 = Index Array(array=w929, index #1=2 ("index"), index #2=0 ("index")) -> (element #1=w926:T44, element #2=w925:T44)
                n459 = control-ref of="This VI"() -> (w924:refnum<vi>)
                n460 = case shown="False" w930 {
                  tunnel: w926 -> [w934 _]
                  tunnel: w925 -> [w933 w945]
                  tunnel: w924 -> [w932 w943]
                  tunnel: T28 {"Left"=0, "Top"=0, "Right"=0, "Bottom"=0} ("Front Panel Window:Window Bounds") -> [w931 w944]
                  frame False {
                    w939 = i16 0
                    n461 = Unbundle By Name(w933) -> ("Bounds.Left"=w936:i16, "Bounds.Bottom"=w937:i16, "Bounds.Top"=w938:i16)
                    n462 = Unbundle By Name(w934) -> ("Bounds.Right"=w935:i16)
                    n463 = Subtract(x=w935, y=w936) -> (x-y=w940:i16)
                    n464 = Subtract(x=w937, y=w938) -> (x-y=w941:i16)
                    n465 = Bundle By Name(cluster=w931, "Left"=w939, "Top"=w939, "Right"=w940, "Bottom"=w941) -> (w942:T28)
                    n466 = property class="VI"(reference=w932, "Front Panel.WinBounds"=w942) -> ()  [unwired: 1 in, 2 out]
                  }
                  frame True {
                    w948 = i16 0
                    n467 = Unbundle By Name(w945) -> ("Bounds.Right"=w951:i16, "Bounds.Bottom"=w950:i16, "Bounds.Top"=w949:i16)
                    n468 = Subtract(x=w950, y=w949) -> (x-y=w947:i16)
                    n469 = Bundle By Name(cluster=w944, "Left"=w948, "Top"=w948, "Right"=w951, "Bottom"=w947) -> (w946:T28)
                    n470 = property class="VI"(reference=w943, "Front Panel.WinBounds"=w946) -> (reference out=w953:refnum<vi>)  [unwired: 1 in, 1 out]
                    n471 = property class="VI"(reference=w953, "FP.State"=T29."Maximized" ("Front Panel Window:State")) -> ()  [unwired: 1 in, 2 out]
                  }
                }
              }
              frame "Add Display" {
                w956 = u16 0 items=["Read", "Write"] ("Action")
                w960 = u16 1 items=["Read", "Write"] ("Action")
                n472 = property on="Add Display" class="Bool (strict)"("Value"=FALSE) -> ()  [unwired: 2 in, 2 out]
                n473 = call "Arange_Displays_V2.vi"("Action"=w956) -> ("Number of Channels OUT"=w957:i32)  [unwired: 14 in]
                n474 = Increment(x=w957) -> (x+1=w959:i32)
                n475 = call "Arange_Displays_V2.vi"("Display References"=w955, "Action"=w960, "Number of Channels"=w959, "Aspect Ratio (h/w)"=1.0) -> ()  [unwired: 11 in, 1 out]
              }
              frame "Remove Display" {
                w963 = u16 0 items=["Read", "Write"] ("Action")
                w967 = u16 1 items=["Read", "Write"] ("Action")
                n476 = call "Arange_Displays_V2.vi"("Action"=w963) -> ("Number of Channels OUT"=w964:i32)  [unwired: 14 in]
                n477 = Decrement(x=w964) -> (x-1=w966:i32)
                n478 = call "Arange_Displays_V2.vi"("Display References"=w962, "Action"=w967, "Number of Channels"=w966, "Aspect Ratio (h/w)"=1.0) -> ()  [unwired: 11 in, 1 out]
                n479 = property on="Remove Display" class="Bool (strict)"("Value"=FALSE) -> ()  [unwired: 2 in, 2 out]
              }
            }
          }
          frame "Graph Tools" {
            n480 = call "Graph_Controls_Ctrl_Index.vi"("OldVal"=w977, "NewVal"=w976) -> ("Control Ref OUT"=w975:refnum<vi>, "Graph Tools Out"=w974:T4)  [unwired: 12 in]
            n481 = property class="Ctl"(reference=w975) -> (reference out=w971:refnum<vi>, "Label.Text"=w970:string)  [unwired: 1 in, 1 out]
            n482 = Unbundle By Name(w974) -> ("Show Cursor"=w973:bool, "Auto Scale"=w972:bool, "Color Map"=w968:T45)
            n483 = case shown="\"Load File\"" w970 {
              selector: w970 -> [_ _ _ w1048 _ _ _ _]
              tunnel: w973 -> [_ w1017 _ _ _ _ _ _]
              tunnel: w972 -> [_ _ w1037 _ _ _ _ _]
              tunnel: w969 -> [w986 w1016 w1038 w1041 w1078 w1099 w1112 w1120]
              tunnel: w971 -> [_ _ _ _ _ _ _ _]
              tunnel: w970 -> [_ _ _ w1043 _ _ _ _]
              tunnel: w968 -> [w989 _ _ _ _ _ _ _]
              frame "Apply Color" {
                n484 = control-ref of="This VI"() -> (w988:refnum<vi>)
                n485 = call "GetDisplayClick.vi"("Display REFs In"=w986, "Calling VI REF"=w988) -> ("Display Index"=w987:i32)  [unwired: 13 in]
                n486 = Index Array(array=w986, index=w987) -> (element=w985:refnum<vi>)
                n487 = property class="IntGraph (strict)"(reference=w985) -> (reference out=w981:refnum<vi>, error out=w978:errorcluster, "ZScale.Maximum"=w984:dbl)  [unwired: 1 in]
                n488 = case shown="\"Gray\"" w989 {
                  tunnel: [cluster{dbl, u32}[] [{0.0, 0}, {0.07843137254901933, 131072}, {0.15686274509805287, 196608}, {0.235294117647058, 327680}, {0.3137254901960773, 458752}, {0.39215686274509665, 589824}, {0.47058823529410176, 720896}, {0.5490196078431353, 851971}, {0.6274509803921546, 983043}, {0.705882352941174, 1114115}, {0.7843137254902075, 1245187}, {0.8627450980392268, 1376259}, {0.941176470588232, 1507331}, {1.0196078431372513, 1638403}, {1.0980392156862848, 1769475}, {1.1764705882353041, 1769479}, {1.2549019607843093, 2031623}, {1.3333333333333286, 2162695}, {1.4117647058823621, 2293767}, {1.4901960784313673, 2424839}, {1.5686274509803866, 2555911}, {1.647058823529406, 2686983}, {1.7254901960784395, 2818055}, {1.8039215686274588, 2949127}, {1.882352941176464, 3080203}, {1.9607843137254832, 3211275}, {2.0392156862745168, 3342347}, {2.117647058823522, 3473419}, {2.1960784313725554, 3604491}, {2.2745098039215605, 3735563}, {2.352941176470594, 3866635}, {2.431372549019599, 3867403}, {2.5098039215686327, 4129547}, {2.588235294117638, 4260619}, {2.6666666666666714, 4391691}, {2.7450980392156907, 4522763}, {2.823529411764696, 4653839}, {2.901960784313715, 4784911}, {2.9803921568627487, 4915983}, {3.058823529411768, 5178127}, {3.1372549019607874, 5309199}, {3.2156862745097925, 5440271}, {3.294117647058826, 5571343}, {3.3725490196078454, 5702415}, {3.4509803921568647, 5703439}, {3.52941176470587, 5965583}, {3.6078431372549034, 6096655}, {3.6862745098039227, 6227727}, {3.764705882352942, 6358799}, {3.8431372549019756, 6489871}, {3.9215686274509807, 6620943}, {4.0, 6752015}, {4.078431372549019, 6883087}, {4.1568627450980244, 7015183}, {4.235294117647058, 7146255}, {4.313725490196077, 7277327}, {4.392156862745097, 7408399}, {4.470588235294102, 7539471}, {4.549019607843135, 7670543}, {4.627450980392155, 7801615}, {4.705882352941174, 8063759}, {4.784313725490179, 8194831}, {4.862745098039213, 8326927}, {4.941176470588232, 8457999}, {5.019607843137251, 8589075}, {5.098039215686285, 8720147}, {5.17647058823529, 8851219}, {5.254901960784309, 8982291}, {5.333333333333329, 9113363}, {5.411764705882362, 9114387}, {5.490196078431367, 9376531}, {5.568627450980401, 9507603}, {5.647058823529406, 9638675}, {5.7254901960784395, 9769747}, {5.803921568627445, 9901843}, {5.882352941176478, 10032915}, {5.960784313725483, 10163987}, {6.039215686274517, 10229523}, {6.117647058823522, 10295059}, {6.196078431372555, 10427155}, {6.2745098039215605, 10558227}, {6.352941176470594, 10689299}, {6.431372549019599, 10820371}, {6.509803921568633, 10886931}, {6.588235294117638, 10952467}, {6.666666666666671, 11083539}, {6.745098039215691, 11214611}, {6.82352941176471, 11215635}, {6.901960784313715, 11477779}, {6.980392156862749, 11543315}, {7.058823529411768, 11608851}, {7.137254901960787, 11740947}, {7.215686274509821, 11806483}, {7.294117647058826, 11872019}, {7.372549019607845, 12004115}, {7.450980392156865, 12135187}, {7.529411764705898, 12266259}, {7.607843137254903, 12267283}, {7.686274509803923, 12398355}, {7.764705882352942, 12529427}, {7.843137254901947, 12530451}, {7.921568627450981, 12595987}, {8.0, 12530451}, {8.07843137254902, 12793619}, {8.156862745098024, 12794131}, {8.235294117647058, 12794643}, {8.313725490196077, 13056787}, {8.392156862745097, 13057299}, {8.47058823529413, 13057811}, {8.549019607843135, 13188883}, {8.627450980392155, 13320979}, {8.705882352941174, 13386515}, {8.784313725490179, 13452563}, {8.862745098039213, 13584147}, {8.941176470588232, 13584659}, {9.019607843137251, 13585171}, {9.098039215686256, 13585683}, {9.17647058823529, 13717267}, {9.254901960784323, 13848339}, {9.333333333333329, 13849363}, {9.411764705882362, 13849875}, {9.490196078431367, 13850387}, {9.5686274509804, 13981459}, {9.647058823529406, 14113555}, {9.72549019607844, 14114067}, {9.803921568627445, 14114579}, {9.882352941176478, 14115091}, {9.960784313725483, 14246675}, {10.039215686274517, 14377747}, {10.117647058823522, 14378771}, {10.196078431372555, 14379283}, {10.27450980392156, 14379539}, {10.352941176470594, 14379795}, {10.4313725490196, 14380819}, {10.509803921568633, 14511891}, {10.588235294117638, 14643987}, {10.666666666666671, 14644503}, {10.745098039215677, 14645015}, {10.82352941176471, 14645527}, {10.901960784313744, 14646039}, {10.980392156862749, 14646551}, {11.058823529411768, 14778135}, {11.137254901960787, 14909207}, {11.215686274509821, 14910231}, {11.294117647058826, 14910747}, {11.372549019607845, 14911259}, {11.450980392156865, 14911771}, {11.52941176470587, 14912283}, {11.607843137254903, 14912797}, {11.686274509803923, 15044383}, {11.764705882352942, 15175455}, {11.843137254901947, 15175967}, {11.92156862745098, 15176479}, {12.0, 15176991}, {12.07843137254902, 15177507}, {12.156862745098053, 15178019}, {12.235294117647058, 15178531}, {12.313725490196092, 15310115}, {12.392156862745097, 15441701}, {12.47058823529413, 15441959}, {12.549019607843135, 15442215}, {12.627450980392155, 15442727}, {12.705882352941174, 15443243}, {12.784313725490179, 15443755}, {12.862745098039213, 15444269}, {12.941176470588246, 15444783}, {13.019607843137251, 15444783}, {13.098039215686285, 15576367}, {13.17647058823529, 15707953}, {13.25490196078431, 15708467}, {13.333333333333329, 15708979}, {13.411764705882362, 15708981}, {13.490196078431367, 15708983}, {13.568627450980387, 15710011}, {13.647058823529406, 15710523}, {13.725490196078411, 15711037}, {13.803921568627459, 15711039}, {13.882352941176464, 15711553}, {13.960784313725512, 15843139}, {14.039215686274517, 15974213}, {14.117647058823522, 15974215}, {14.196078431372541, 15974217}, {14.27450980392156, 15974219}, {14.352941176470594, 15975755}, {14.431372549019613, 15976271}, {14.509803921568633, 15976785}, {14.588235294117666, 15977299}, {14.666666666666671, 15977301}, {14.745098039215677, 15977815}, {14.82352941176471, 15978327}, {14.901960784313744, 15978331}, {14.980392156862749, 16109917}, {15.058823529411768, 16241503}, {15.137254901960787, 16241505}, {15.215686274509792, 16242019}, {15.294117647058826, 16242535}, {15.372549019607845, 16242537}, {15.450980392156865, 16242539}, {15.529411764705898, 16243563}, {15.607843137254903, 16243567}, {15.686274509803908, 16244081}, {15.764705882352942, 16244595}, {15.843137254901947, 16244599}, {15.92156862745098, 16244601}, {16.0, 16244603}, {16.07843137254902, 16245627}, {16.156862745098024, 16245631}, {16.235294117647058, 16245633}, {16.313725490196077, 16246147}, {16.392156862745097, 16246663}, {16.47058823529413, 16377735}, {16.549019607843135, 16508811}, {16.62745098039217, 16508815}, {16.705882352941174, 16509839}, {16.78431372549018, 16509843}, {16.862745098039213, 16509845}, {16.941176470588232, 16509847}, {17.01960784313725, 16510361}, {17.098039215686256, 16510875}, {17.17647058823529, 16510879}, {17.25490196078431, 16510881}, {17.33333333333333, 16510883}, {17.411764705882362, 16511399}, {17.49019607843138, 16511911}, {17.568627450980387, 16511915}, {17.647058823529406, 16511917}, {17.72549019607844, 16511919}, {17.80392156862746, 16511923}, {17.882352941176464, 16512437}, {17.960784313725483, 16512951}, {18.03921568627449, 16512955}, {18.117647058823522, 16512957}, {18.19607843137254, 16512959}, {18.27450980392156, 16512961}, {18.352941176470594, 16512963}, {18.431372549019613, 16512967}, {18.509803921568633, 16513481}, {18.588235294117638, 16513995}, {18.66666666666667, 16513999}, {18.74509803921569, 16514001}, {18.82352941176471, 16514003}, {18.901960784313744, 16514005}, {18.98039215686275, 16514007}, {19.058823529411754, 16514011}, {19.137254901960787, 16514013}, {19.215686274509792, 16514015}, {19.294117647058826, 16514019}, {19.372549019607845, 16514021}, {19.450980392156865, 16514023}, {19.52941176470587, 16514027}, {19.607843137254918, 16514029}, {19.686274509803923, 16514031}, {19.764705882352942, 16514035}, {19.843137254901947, 16514037}, {19.921568627450995, 16514039}, {20.0, 16514043}] ("Z Scale.Marker Values[]") cluster{dbl, u32}[] [{0.0, 0}, {85.0, 16711680}, {108.0, 16729344}, {127.0, 16744192}, {132.0, 16747520}, {140.0, 16753920}, {157.0, 16766720}, {170.0, 16776960}, {245.0, 16777184}, {250.0, 16777200}, {255.0, 16777215}] ("Z Scale.Marker Values[]") cluster{dbl, u32}[] [{0.0, 0}, {255.0, 16777215}] ("Z Scale.Marker Values[]") cluster{dbl, u32}[] [{0.0, 0}, {255.0, 16711680}] ("Z Scale.Marker Values[]") cluster{dbl, u32}[] [{0.0, 0}, {255.0, 65280}] ("Z Scale.Marker Values[]") cluster{dbl, u32}[] [{0.0, 0}, {255.0, 255}] ("Z Scale.Marker Values[]") cluster{dbl, u32}[] [{0.0, 0}, {255.0, 65535}] ("Z Scale.Marker Values[]") cluster{dbl, u32}[] [{0.0, 0}, {255.0, 16711935}] ("Z Scale.Marker Values[]") cluster{dbl, u32}[] [{0.0, 0}, {255.0, 16776960}] ("Z Scale.Marker Values[]") cluster{dbl, u32}[] [{0.0, 0}, {170.0, 16711680}, {245.0, 16777184}, {250.0, 16777200}, {255.0, 16448250}] ("Z Scale.Marker Values[]") cluster{dbl, u32}[] [{0.0, 0}, {170.0, 65280}, {245.0, 16777184}, {250.0, 16777200}, {255.0, 16448250}] ("Z Scale.Marker Values[]") cluster{dbl, u32}[] [{0.0, 0}, {170.0, 255}, {245.0, 16777184}, {250.0, 16777200}, {255.0, 16448250}] ("Z Scale.Marker Values[]") cluster{dbl, u32}[] [{0.0, 0}, {1.0, 131072}, {2.0, 196608}, {3.0, 327680}, {4.0, 458752}, {5.0, 589824}, {6.0, 720896}, {7.0, 851971}, {8.0, 983043}, {9.0, 1114115}, {10.0, 1245187}, {11.0, 1376259}, {12.0, 1507331}, {13.0, 1638403}, {14.0, 1769475}, {15.0, 1769479}, {16.0, 2031623}, {17.0, 2162695}, {18.0, 2293767}, {19.0, 2424839}, {20.0, 2555911}, {21.0, 2686983}, {22.0, 2818055}, {23.0, 2949127}, {24.0, 3080203}, {25.0, 3211275}, {26.0, 3342347}, {27.0, 3473419}, {28.0, 3604491}, {29.0, 3735563}, {30.0, 3866635}, {31.0, 3867403}, {32.0, 4129547}, {33.0, 4260619}, {34.0, 4391691}, {35.0, 4522763}, {36.0, 4653839}, {37.0, 4784911}, {38.0, 4915983}, {39.0, 5178127}, {40.0, 5309199}, {41.0, 5440271}, {42.0, 5571343}, {43.0, 5702415}, {44.0, 5703439}, {45.0, 5965583}, {46.0, 6096655}, {47.0, 6227727}, {48.0, 6358799}, {49.0, 6489871}, {50.0, 6620943}, {51.0, 6752015}, {52.0, 6883087}, {53.0, 7015183}, {54.0, 7146255}, {55.0, 7277327}, {56.0, 7408399}, {57.0, 7539471}, {58.0, 7670543}, {59.0, 7801615}, {60.0, 8063759}, {61.0, 8194831}, {62.0, 8326927}, {63.0, 8457999}, {64.0, 8589075}, {65.0, 8720147}, {66.0, 8851219}, {67.0, 8982291}, {68.0, 9113363}, {69.0, 9114387}, {70.0, 9376531}, {71.0, 9507603}, {72.0, 9638675}, {73.0, 9769747}, {74.0, 9901843}, {75.0, 10032915}, {76.0, 10163987}, {77.0, 10229523}, {78.0, 10295059}, {79.0, 10427155}, {80.0, 10558227}, {81.0, 10689299}, {82.0, 10820371}, {83.0, 10886931}, {84.0, 10952467}, {85.0, 11083539}, {86.0, 11214611}, {87.0, 11215635}, {88.0, 11477779}, {89.0, 11543315}, {90.0, 11608851}, {91.0, 11740947}, {92.0, 11806483}, {93.0, 11872019}, {94.0, 12004115}, {95.0, 12135187}, {96.0, 12266259}, {97.0, 12267283}, {98.0, 12398355}, {99.0, 12529427}, {100.0, 12530451}, {101.0, 12595987}, {102.0, 12530451}, {103.0, 12793619}, {104.0, 12794131}, {105.0, 12794643}, {106.0, 13056787}, {107.0, 13057299}, {108.0, 13057811}, {109.0, 13188883}, {110.0, 13320979}, {111.0, 13386515}, {112.0, 13452563}, {113.0, 13584147}, {114.0, 13584659}, {115.0, 13585171}, {116.0, 13585683}, {117.0, 13717267}, {118.0, 13848339}, {119.0, 13849363}, {120.0, 13849875}, {121.0, 13850387}, {122.0, 13981459}, {123.0, 14113555}, {124.0, 14114067}, {125.0, 14114579}, {126.0, 14115091}, {127.0, 14246675}, {128.0, 14377747}, {129.0, 14378771}, {130.0, 14379283}, {131.0, 14379539}, {132.0, 14379795}, {133.0, 14380819}, {134.0, 14511891}, {135.0, 14643987}, {136.0, 14644503}, {137.0, 14645015}, {138.0, 14645527}, {139.0, 14646039}, {140.0, 14646551}, {141.0, 14778135}, {142.0, 14909207}, {143.0, 14910231}, {144.0, 14910747}, {145.0, 14911259}, {146.0, 14911771}, {147.0, 14912283}, {148.0, 14912797}, {149.0, 15044383}, {150.0, 15175455}, {151.0, 15175967}, {152.0, 15176479}, {153.0, 15176991}, {154.0, 15177507}, {155.0, 15178019}, {156.0, 15178531}, {157.0, 15310115}, {158.0, 15441701}, {159.0, 15441959}, {160.0, 15442215}, {161.0, 15442727}, {162.0, 15443243}, {163.0, 15443755}, {164.0, 15444269}, {165.0, 15444783}, {166.0, 15444783}, {167.0, 15576367}, {168.0, 15707953}, {169.0, 15708467}, {170.0, 15708979}, {171.0, 15708981}, {172.0, 15708983}, {173.0, 15710011}, {174.0, 15710523}, {175.0, 15711037}, {176.0, 15711039}, {177.0, 15711553}, {178.0, 15843139}, {179.0, 15974213}, {180.0, 15974215}, {181.0, 15974217}, {182.0, 15974219}, {183.0, 15975755}, {184.0, 15976271}, {185.0, 15976785}, {186.0, 15977299}, {187.0, 15977301}, {188.0, 15977815}, {189.0, 15978327}, {190.0, 15978331}, {191.0, 16109917}, {192.0, 16241503}, {193.0, 16241505}, {194.0, 16242019}, {195.0, 16242535}, {196.0, 16242537}, {197.0, 16242539}, {198.0, 16243563}, {199.0, 16243567}, {200.0, 16244081}, {201.0, 16244595}, {202.0, 16244599}, {203.0, 16244601}, {204.0, 16244603}, {205.0, 16245627}, {206.0, 16245631}, {207.0, 16245633}, {208.0, 16246147}, {209.0, 16246663}, {210.0, 16377735}, {211.0, 16508811}, {212.0, 16508815}, {213.0, 16509839}, {214.0, 16509843}, {215.0, 16509845}, {216.0, 16509847}, {217.0, 16510361}, {218.0, 16510875}, {219.0, 16510879}, {220.0, 16510881}, {221.0, 16510883}, {222.0, 16511399}, {223.0, 16511911}, {224.0, 16511915}, {225.0, 16511917}, {226.0, 16511919}, {227.0, 16511923}, {228.0, 16512437}, {229.0, 16512951}, {230.0, 16512955}, {231.0, 16512957}, {232.0, 16512959}, {233.0, 16512961}, {234.0, 16512963}, {235.0, 16512967}, {236.0, 16513481}, {237.0, 16513995}, {238.0, 16513999}, {239.0, 16514001}, {240.0, 16514003}, {241.0, 16514005}, {242.0, 16514007}, {243.0, 16514011}, {244.0, 16514013}, {245.0, 16514015}, {246.0, 16514019}, {247.0, 16514021}, {248.0, 16514023}, {249.0, 16514027}, {250.0, 16514029}, {251.0, 16514031}, {252.0, 16514035}, {253.0, 16514037}, {254.0, 16514039}, {255.0, 16514043}] ("Z Scale.Marker Values[]")] -> w980
                  tunnel: w984 -> [w991 w992 w994 w996 w998 w1000 w1002 w1004 w1006 w1008 w1010 w1012 w1015]
                  tunnel: [w991 w992 w994 w996 w998 w1000 w1002 w1004 w1006 w1008 w1010 w1012 w1015] -> w982
                  frame "System", Default {
                  }
                  frame "Fire" {
                    # "Fire"
                  }
                  frame "Gray" {
                    # "Grayscale"
                  }
                  frame "Red" {
                    # "Red"
                  }
                  frame "Green" {
                    # "Green"
                  }
                  frame "Blue" {
                    # "Blue"
                  }
                  frame "Cyan" {
                    # "Cyan"
                  }
                  frame "Magenta" {
                    # "Magenta"
                  }
                  frame "Yellow" {
                    # "Yellow"
                  }
                  frame "Red-White" {
                    # "Red-White"
                  }
                  frame "Green-White" {
                    # "Green-White"
                  }
                  frame "Blue-White" {
                    # "Blue-White"
                  }
                  frame "Glow" {
                  }
                }
                n489 = property on="Apply Color" class="Bool (strict)"(error in=w978, "Value"=FALSE) -> ()  [unwired: 1 in, 2 out]
                n490 = property class="IntGraph (strict)"(reference=w981, "ZScale.MarkerVals[]"=w980, "ZScale.High Color"=u32 255, "ZScale.Maximum"=w982) -> ()  [unwired: 1 in, 2 out]
              }
              frame "Show Cursor", Default {
                w1020 = 2.0 ("y")
                n491 = Index Array(array=w1016, index=0) -> (element=w1028:refnum<vi>)
                n492 = property class="IntGraph (strict)"(reference=w1028) -> ("Value"=w1027:sgl[][])  [unwired: 1 in, 2 out]
                n493 = Array Size(array=w1027) -> (size(s)=w1026:i32[])
                n494 = To Double Precision Float(number=w1026) -> (double precision float=w1023:dbl[])
                n495 = Index Array(array=w1023, index #1=0 ("index"), index #2=1 ("index")) -> (element #1=w1022:dbl, element #2=w1021:dbl)
                n496 = Divide(x=w1022, y=w1020) -> (x/y=w1019:dbl)
                n497 = Divide(x=w1021, y=w1020) -> (x/y=w1018:dbl)
                n498 = for {
                  tunnel: w1016 -> [w1030] mode=indexing
                  tunnel: w1019 -> [w1032]
                  tunnel: w1018 -> [w1031]
                  tunnel: w1017 -> [w1033]
                  n499 = property class="IntGraph (strict)"(reference=w1030, "Cursor.Visible"=w1033, "Cursor.Cursor X"=w1032, "Cursor.Cursor Y"=w1031) -> ()  [unwired: 1 in, 2 out]
                }
              }
              frame "Auto Scale" {
                n500 = Select(t=u8 2 ("Z Scale.Scale Fit"), s=w1037, f=u8 0) -> (s? t:f=w1034:u8)
                n501 = for {
                  tunnel: w1038 -> [w1040] mode=indexing
                  tunnel: w1034 -> [w1039]
                  n502 = property class="IntGraph (strict)"(reference=w1040, "ZScale.ScaleFit"=w1039) -> ()  [unwired: 1 in, 2 out]
                }
              }
              frame "Pan Tool", "Reset Zoom", "Zoom In", "Zoom Out" {
                n503 = case shown="\"Reset Zoom\"" w1048 {
                  tunnel: [0 ("Palette:Active Tool") 6 ("Palette:Active Tool") 7 ("Palette:Active Tool") 1 ("Palette:Active Tool") 0 ("Palette:Active Tool")] -> w1042
                  tunnel: w1041 -> [_ _ _ _ w1060]
                  frame Default {
                  }
                  frame "Zoom In" {
                  }
                  frame "Zoom Out" {
                  }
                  frame "Pan Tool" {
                  }
                  frame "Reset Zoom" {
                    n504 = property on="Reset Zoom" class="Bool (strict)"("Value"=FALSE) -> ()  [unwired: 2 in, 2 out]
                    n505 = for {
                      tunnel: w1060 -> [w1065] mode=indexing
                      tunnel: 5 ("Palette:Active Tool") -> [w1064]
                      n506 = property class="IntGraph (strict)"(reference=w1065, "ActPaletteTool"=w1064) -> ()  [unwired: 1 in, 2 out]
                    }
                  }
                }
                n507 = control-ref of="Zoom In"() -> (w1044:refnum<vi>)
                n508 = control-ref of="Zoom Out"() -> (w1046:refnum<vi>)
                n509 = control-ref of="Pan Tool"() -> (w1045:refnum<vi>)
                n510 = Build Array(w1044, w1046, w1045) -> (w1047:refnum<vi>[])
                n511 = for {
                  tunnel: w1047 -> [w1053] mode=indexing
                  tunnel: w1043 -> [w1051]
                  n512 = property class="Bool (strict)"(reference=w1053) -> (reference out=w1052:refnum<vi>, "Label.Text"=w1050:string)  [unwired: 1 in, 1 out]
                  n513 = Equal?(x=w1050, y=w1051) -> (x = y?=w1049:bool)
                  n514 = property class="Bool (strict)"(reference=w1052, "Value"=w1049) -> ()  [unwired: 1 in, 2 out]
                }
                n515 = for {
                  tunnel: w1041 -> [w1055] mode=indexing
                  tunnel: w1042 -> [w1054]
                  n516 = property class="IntGraph (strict)"(reference=w1055, "ActPaletteTool"=w1054) -> ()  [unwired: 1 in, 2 out]
                }
              }
              frame "Load File" {
                w1075 = u16 1 items=["Get Image", "Load and Read File"] ("Action")
                n517 = control-ref of="This VI"() -> (w1077:refnum<vi>)
                n518 = property on="Load File" class="Bool (strict)"("Value"=FALSE) -> ()  [unwired: 2 in, 2 out]
                n519 = call "GetDisplayClick.vi"("Display REFs In"=w1078, "Calling VI REF"=w1077) -> ("Display Index"=w1071:i32)  [unwired: 13 in]
                n520 = call "OpenDBL.vi"("Action"=w1075) -> ("Image"=w1068:sgl[], "Dimensions (Z, Y, X, t)"=w1074:i32[])  [unwired: 11 in, 2 out]
                n521 = Index Array(array=w1074, index #1=1 ("index"), index #2=2 ("index")) -> (element #1=w1067:i32, element #2=w1066:i32)
                n522 = case shown="Default" w1071 {
                  selector: w1071 -> [w1084 w1093]
                  tunnel: [w1084 w1093] -> w1070
                  tunnel: [w1080 w1085] -> w1069
                  tunnel: w1068 -> [w1083 w1092]
                  tunnel: w1067 -> [w1082 w1091]
                  tunnel: w1066 -> [w1081 w1090]
                  frame 0, 1 {
                    n523 = Reshape Array(w1083, w1082, w1081) -> (w1080:sgl[][])
                  }
                  frame Default {
                    n524 = Reshape Array(w1092, w1091, w1090) -> (w1089:sgl[][])
                    n525 = call "ArrayTransformations.vi"("Input"=w1089, "Option"="Rotate 90") -> ("Output"=w1087:sgl[][])
                    n526 = call "ArrayTransformations.vi"("Input"=w1087, "Option"="Horizontal Flip") -> ("Output"=w1085:sgl[][])
                  }
                }
                n527 = Index Array(array=w1078, index=w1070) -> (element=w1076:refnum<vi>)
                n528 = property class="IntGraph (strict)"(reference=w1076, "Value"=w1069) -> ()  [unwired: 1 in, 2 out]
              }
              frame "Fit Tool" {
                n529 = control-ref of="This VI"() -> (w1101:refnum<vi>)
                n530 = call "Image Aquisition Param Ctrl_AE.vi"("Action"=enum16{"READ", "WRITE"}."READ") -> ("Image Acquisition Parameters Out"=w1096:T19)  [unwired: 10 in]
                n531 = call "GetDisplayClick.vi"("Display REFs In"=w1099, "Calling VI REF"=w1101) -> ("Display Index"=w1100:i32)  [unwired: 13 in]
                n532 = Index Array(array=w1099, index=w1100) -> (element=w1098:refnum<vi>)
                n533 = property class="IntGraph (strict)"(reference=w1098) -> ("Value"=w1097:sgl[][])  [unwired: 1 in, 2 out]
                n534 = vi-ref "QuickProfile_V3.vi"() -> (w1104:refnum<vi>)
                n535 = property class="VI Interface Type 0"(reference=w1104) -> ("Path"=w1107:path)  [unwired: 1 in, 2 out]
                n536 = Unbundle By Name(w1096) -> ("Pixel Size (nm)"=w1103:dbl[])
                n537 = Index Array(array=w1103, index=0) -> (element=w1110:dbl)
                n538 = Open VI Reference(type specifier VI Refnum (for type only)=w1104, vi path=w1107, options=128) -> (vi reference=w1105:refnum<vi>)  [unwired: 3 in, 1 out]
                n539 = call-by-ref "Start Asynchronous Call"(reference=w1105, "Image IN"=w1097, "Pixel Size (nm)"=w1110) -> (reference out=w1108:refnum<vi>, error out=w1095:errorcluster)  [unwired: 15 in]
                n540 = Close Reference(reference=w1108) -> ()  [unwired: 1 in, 1 out]
                n541 = property on="Fit Tool" class="Bool (strict)"(error in=w1095, "Value"=FALSE) -> ()  [unwired: 1 in, 2 out]
              }
              frame "Smooth Tool" {
                n542 = vi-ref "SmoothTool.vi"() -> (w1115:refnum<vi>)
                n543 = property on="Smooth Tool" class="Bool (strict)"("Value"=FALSE) -> ()  [unwired: 2 in, 2 out]
                n544 = property class="VI Interface Type 1"(reference=w1115) -> ("Path"=w1117:path)  [unwired: 1 in, 2 out]
                n545 = control-ref of="This VI"() -> (w1113:refnum<vi>)
                n546 = Open VI Reference(type specifier VI Refnum (for type only)=w1115, vi path=w1117, options=128) -> (vi reference=w1116:refnum<vi>)  [unwired: 3 in, 1 out]
                n547 = call-by-ref "Start Asynchronous Call"(reference=w1116, "Calling VI REF"=w1113, "Display REFs In"=w1112) -> (reference out=w1114:refnum<vi>)  [unwired: 11 in, 1 out]
                n548 = Close Reference(reference=w1114) -> ()  [unwired: 1 in, 1 out]
              }
              frame "Merge Tool" {
                n549 = vi-ref "MergeTool - Cambridge.vi"() -> (w1123:refnum<vi>)
                n550 = property class="VI Interface Type 2"(reference=w1123) -> ("Path"=w1125:path)  [unwired: 1 in, 2 out]
                n551 = property on="Merge Tool" class="Bool (strict)"("Value"=FALSE) -> ()  [unwired: 2 in, 2 out]
                n552 = control-ref of="This VI"() -> (w1121:refnum<vi>)
                n553 = Open VI Reference(type specifier VI Refnum (for type only)=w1123, vi path=w1125, options=128) -> (vi reference=w1124:refnum<vi>)  [unwired: 3 in, 1 out]
                n554 = call-by-ref "Start Asynchronous Call"(reference=w1124, "VI Reference"=w1121, "Display References"=w1120) -> (reference out=w1122:refnum<vi>)  [unwired: 11 in, 1 out]
                n555 = Close Reference(reference=w1122) -> ()  [unwired: 1 in, 1 out]
              }
            }
          }
        }
      }
      event "Channel 1", "Channel 2", "Channel 3", "Channel 4", "Channel 5", "Channel 6": Mouse Down; "Channel 1", "Channel 2", "Channel 3", "Channel 4", "Channel 5", "Channel 6": Mouse Up {
        n556 = event-data() -> ("Type"=w1132:T30, "CtlRef"=w1129:refnum<vi>)  [unwired: 1 in, 5 out]
        n557 = Equal?(x=w1132, y=lveventtype."Mouse Down" ("Type")) -> (x = y?=w1130:bool)
        n558 = call "Graph Ref AE.vi"("Action"=enum16{"READ", "WRITE"}."READ") -> ("Graph Ref Out"=w1127:refnum<vi>[])  [unwired: 10 in]
        n559 = case shown="True" w1130 {
          tunnel: w1129 -> [w1135 w1153]
          tunnel: w1127 -> [w1134 w1152]
          frame False {
            n560 = property class="IntGraph (strict)"(reference=w1135) -> (reference out=w1139:refnum<vi>, "ActPaletteTool"=w1136:i32)  [unwired: 1 in, 1 out]
            n561 = Not Equal?(x=w1136, y=0) -> (x != y?=w1138:bool)
            n562 = case shown="False" w1138 {
              tunnel: w1139 -> [w1142 w1148]
              tunnel: w1134 -> [w1141 w1145]
              frame False {
                n563 = property class="IntGraph (strict)"(reference=w1142) -> ("Cursor.Cursor Position"=w1140:T46)  [unwired: 1 in, 2 out]
                n564 = for {
                  tunnel: w1141 -> [w1143] mode=indexing
                  tunnel: w1140 -> [w1144]
                  n565 = property class="IntGraph (strict)"(reference=w1143, "Cursor.Cursor Position"=w1144) -> ()  [unwired: 1 in, 2 out]
                }
              }
              frame True {
                n566 = property class="IntGraph (strict)"(reference=w1148) -> ("XScale.Range"=w1147:T47, "YScale.Range"=w1146:T47)  [unwired: 1 in, 2 out]
                n567 = for {
                  tunnel: w1147 -> [w1151]
                  tunnel: w1146 -> [w1150]
                  tunnel: w1145 -> [w1149] mode=indexing
                  n568 = property class="IntGraph (strict)"(reference=w1149, "XScale.Range"=w1151, "YScale.Range"=w1150) -> ()  [unwired: 1 in, 2 out]
                }
              }
            }
          }
          frame True {
            n569 = for {
              tunnel: w1152 -> [w1158] mode=indexing
              tunnel: w1153 -> [w1159]
              n570 = Equal?(x=w1158, y=w1159) -> (x = y?=w1157:bool)
              n571 = Select(t=T31 {"Left"=2431, "Top"=-324} ("Z Scale.Position"), s=w1157, f=T31 {"Left"=0, "Top"=0}) -> (s? t:f=w1154:T31)
              n572 = property class="IntGraph (strict)"(reference=w1158, "ZScale.Visible"=w1157, "ZScale.Position"=w1154) -> ()  [unwired: 1 in, 2 out]
            }
          }
        }
      }
      event "Wake Up FPGA", "Follow Cursor": Value Change {
        n573 = event-data() -> ("CtlRef"=w1163:refnum<vi>, "NewVal"=w1161:bool)  [unwired: 1 in]
        n574 = property class="Bool"(reference=w1163) -> ("Label.Text"=w1162:string)  [unwired: 1 in, 2 out]
        n575 = case shown="\"Follow Cursor\", Default" w1162 {
          tunnel: w1161 -> [w1165 _]
          frame "Follow Cursor", Default {
            n576 = control-ref of="Channel 1"() -> (w1164:refnum<vi>)
            n577 = case shown="True" w1165 {
              tunnel: w1164 -> [w1170 w1175]
              frame False {
                n578 = property class="IntGraph (strict)"(reference=w1170, "Active Cursor"=u32 1, "Cursor.Visible"=FALSE) -> (reference out=w1166:refnum<vi>)  [unwired: 1 in, 1 out]
                n579 = flat-sequence {
                  frame #0 {
                    n580 = call "Galvo Offset AE v1.vi"("Galvo 1 Offset In"=-0.15, "Action"=enum16{"Read", "Write"}."Write") -> ()  [unwired: 2 out]
                  }
                  frame #1 {
                    n581 = call "FPGA-7842R-Control V2.vi"("Action"=FPGA-7842R-Reference."Set Galvo", "Initialize"=TRUE) -> ()  [unwired: 12 in, 2 out]
                  }
                }
                n582 = property class="IntGraph (strict)"(reference=w1166, "Active Cursor"=u32 0) -> ()  [unwired: 1 in, 2 out]
              }
              frame True {
                # "open independent VI to set the offset"
                n583 = vi-ref "Set Position AE.vi"() -> (w1181:refnum<vi>)
                n584 = property class="VI Interface Type 3"(reference=w1181) -> ("Path"=w1182:path)  [unwired: 1 in, 2 out]
                n585 = Open VI Reference(type specifier VI Refnum (for type only)=w1181, vi path=w1182, options=128) -> (vi reference=w1184:refnum<vi>)  [unwired: 3 in, 1 out]
                n586 = call-by-ref "?"(reference=w1184) -> (reference out=w1180:refnum<vi>, "Cursor Y"=w1177:dbl)  [unwired: 2 in, 1 out]
                n587 = Close Reference(reference=w1180) -> ()  [unwired: 1 in, 1 out]
                n588 = property class="IntGraph (strict)"(reference=w1175, "Active Cursor"=u32 1, "Cursor.Visible"=TRUE, "Cursor.Cursor X"=-1.0 ("Cursor.Cursor Position:Cursor X"), "Cursor.Cursor Y"=w1177) -> ()  [unwired: 1 in, 2 out]
              }
            }
          }
          frame "Wake Up FPGA" {
            n589 = flat-sequence {
              frame #0 {
                n590 = xnode "Open FPGA VI Reference"() -> ("FPGA VI Reference Out"=w1186:refnum<k20>, "error out"=w1185:errorcluster)  [unwired: 2 in]
                n591 = xnode "Invoke Method"("FPGA VI Reference In"=w1186, "error in"=w1185) -> ()  [unwired: 2 out]
              }
              frame #1 {
                n592 = call "FPGA-7842R-Control V2.vi"("Action"=FPGA-7842R-Reference."Initialize", "Initialize"=FALSE) -> ()  [unwired: 12 in, 2 out]
              }
              frame #2 {
                n593 = One Button Dialog(message="FPGA is reinitialized!") -> ()  [unwired: 1 in, 1 out]
              }
            }
          }
        }
      }
      event "Sequence Cluster": Value Change {
        n594 = event-data() -> ("CtlRef"=w1193:refnum<vi>, "OldVal"=w1197:T15, "NewVal"=w1196:T15)  [unwired: 1 in]
        n595 = Not Equal?(x=w1197, y=w1196) -> (x != y?=w1195:T48)
        n596 = property class="Clust"(reference=w1193) -> ("Controls[]"=w1192:refnum<vi>[])  [unwired: 1 in, 2 out]
        n597 = Cluster To Array(cluster=w1195) -> (array=w1194:bool[])
        n598 = for {
          tunnel: w1194 -> [w1198] mode=indexing
          tunnel: w1192 -> [w1199] mode=indexing
          tunnel: [w1199] -> w1191
          stop <- w1198 stop-if-true
        }
        n599 = property class="Ctl"(reference=w1191) -> ("Label.Text"=w1190:string)  [unwired: 1 in, 2 out]
        n600 = case shown="\"DeleteSeq\"" w1190 {
          frame Default {
          }
          frame "Sequence List" {
            w1200 = enum16{"READ", "WRITE"}."WRITE" ("Action")
            n601 = property on="Sequence List" class="RadioBtnsControl (strict)"() -> ("Value"=w1205:enum32{"Seq 1", "Seq 2", "Seq 3", "Seq 4"})  [unwired: 2 in, 2 out]
            n602 = call "Seq AE.vi"("Action"=enum16{"READ", "BUILD", "WRITE", "DELETE"}."READ") -> ("Array"=w1206:T39)  [unwired: 8 in]
            n603 = Index Array(array=w1206, index=w1205) -> (element=w1204:T40)
            n604 = Unbundle By Name(w1204) -> ("Detectors Parameters Out"=w1203:T17, "Laser Parameters Out"=w1202:T18, "Image Acquisition Parameters Out"=w1201:T19)
            n605 = call "Detectors Crl_AE.vi"("Action"=w1200, "Detectors Parameters In"=w1203) -> ()  [unwired: 9 in, 1 out]
            n606 = call "LASERs_ Crl_AE.vi"("Action"=w1200, "Laser Parameters In"=w1202) -> ()  [unwired: 9 in, 1 out]
            n607 = call "Image Aquisition Param Ctrl_AE.vi"("Action"=w1200, "Image Acquisition Parameters In"=w1201) -> ()  [unwired: 9 in, 1 out]
          }
          frame "Operation Option" {
          }
          frame "AddSeq" {
            n608 = call "LASERs_ Crl_AE.vi"("Action"=enum16{"READ", "WRITE"}."READ") -> ("Laser Parameters Out"=w1212:T18)  [unwired: 10 in]
            n609 = call "Detectors Crl_AE.vi"("Action"=enum16{"READ", "WRITE"}."READ") -> ("Detectors Parameters Out"=w1213:T17)  [unwired: 10 in]
            n610 = call "Image Aquisition Param Ctrl_AE.vi"("Action"=enum16{"READ", "WRITE"}."READ") -> ("Image Acquisition Parameters Out"=w1211:T19)  [unwired: 10 in]
            n611 = Bundle("Detectors Parameters Out"=w1213, "Laser Parameters Out"=w1212, "Image Acquisition Parameters Out"=w1211) -> (w1209:T40)  [unwired: 1 in]
            n612 = property on="Sequence List" class="RadioBtnsControl (strict)"() -> ("DisabledEnum"=w1210:T25)  [unwired: 2 in, 2 out]
            n613 = case shown="\"Disabled\", \"Disabled and Grayed Out\", Default" w1210 {
              tunnel: [enum16{"READ", "BUILD", "WRITE", "DELETE"}."BUILD" ("Action") w1223] -> w1208
              frame "Disabled", "Disabled and Grayed Out", Default {
                w1218 = T25."Enabled" ("Disabled")
                n614 = property on="Sequence List" class="RadioBtnsControl (strict)"("DisabledEnum"=w1218) -> ()  [unwired: 2 in, 2 out]
                n615 = property on="Seq 1" class="Bool (strict)"("DisabledEnum"=w1218) -> ()  [unwired: 2 in, 2 out]
                n616 = property on="Seq 1" class="Bool (strict)"("Value"=TRUE) -> ()  [unwired: 2 in, 2 out]
              }
              frame "Enabled" {
                n617 = call "Seq AE.vi"("Action"=enum16{"READ", "BUILD", "WRITE", "DELETE"}."READ") -> ("Array"=w1221:T39)  [unwired: 8 in]
                n618 = Array Size(array=w1221) -> (size(s)=w1220:i32)
                n619 = case shown="1" w1220 {
                  tunnel: [enum16{"READ", "BUILD", "WRITE", "DELETE"}."READ" ("Action") enum16{"READ", "BUILD", "WRITE", "DELETE"}."WRITE" ("Action") enum16{"READ", "BUILD", "WRITE", "DELETE"}."WRITE" ("Action") enum16{"READ", "BUILD", "WRITE", "DELETE"}."WRITE" ("Action")] -> w1223
                  frame 4, Default {
                    n620 = One Button Dialog(message="No more sequence allowed!") -> ()  [unwired: 1 in, 1 out]
                  }
                  frame 1 {
                    n621 = property on="Seq 2" class="Bool (strict)"("DisabledEnum"=T25."Enabled" ("Disabled")) -> ()  [unwired: 2 in, 2 out]
                    n622 = property on="Seq 2" class="Bool (strict)"("Value"=TRUE) -> ()  [unwired: 2 in, 2 out]
                  }
                  frame 2 {
                    n623 = property on="Seq 3" class="Bool (strict)"("DisabledEnum"=T25."Enabled" ("Disabled")) -> ()  [unwired: 2 in, 2 out]
                    n624 = property on="Seq 3" class="Bool (strict)"("Value"=TRUE) -> ()  [unwired: 2 in, 2 out]
                  }
                  frame 3 {
                    n625 = property on="Seq 4" class="Bool (strict)"("DisabledEnum"=T25."Enabled" ("Disabled")) -> ()  [unwired: 2 in, 2 out]
                    n626 = property on="Seq 4" class="Bool (strict)"("Value"=TRUE) -> ()  [unwired: 2 in, 2 out]
                  }
                }
              }
            }
            n627 = call "Seq AE.vi"("Action"=w1208, "Cluster"=w1209) -> ()  [unwired: 7 in, 1 out]
          }
          frame "DeleteSeq" {
            n628 = call "Seq AE.vi"("Action"=enum16{"READ", "BUILD", "WRITE", "DELETE"}."READ") -> ("Array"=w1236:T39)  [unwired: 8 in]
            n629 = Array Size(array=w1236) -> (size(s)=w1235:i32)
            n630 = case shown="2..4" w1235 {
              selector: w1235 -> [_ _ w1241]
              frame 0, Default {
              }
              frame 1 {
                n631 = call "Seq AE.vi"("Action"=enum16{"READ", "BUILD", "WRITE", "DELETE"}."DELETE") -> ()  [unwired: 8 in, 1 out]
                n632 = property on="Sequence List" class="RadioBtnsControl (strict)"("DisabledEnum"=T25."Disabled and Grayed Out" ("Disabled")) -> ()  [unwired: 2 in, 2 out]
              }
              frame 2..4 {
                n633 = property on="Sequence List" class="RadioBtnsControl (strict)"() -> ("Value"=w1243:enum32{"Seq 1", "Seq 2", "Seq 3", "Seq 4"})  [unwired: 2 in, 2 out]
                n634 = Decrement(x=w1241) -> (x-1=w1242:i32)
                n635 = Equal?(x=w1242, y=w1243) -> (x = y?=w1244:bool)
                n636 = call "Seq AE.vi"("Action"=enum16{"READ", "BUILD", "WRITE", "DELETE"}."DELETE") -> ("Array"=w1240:T39)  [unwired: 8 in]
                n637 = case shown="4" w1241 {
                  frame 2, Default {
                    n638 = property on="Seq 2" class="Bool (strict)"("DisabledEnum"=T25."Disabled and Grayed Out" ("Disabled")) -> ()  [unwired: 2 in, 2 out]
                  }
                  frame 3 {
                    n639 = property on="Seq 3" class="Bool (strict)"("DisabledEnum"=T25."Disabled and Grayed Out" ("Disabled")) -> ()  [unwired: 2 in, 2 out]
                  }
                  frame 4 {
                    n640 = property on="Seq 4" class="Bool (strict)"("DisabledEnum"=T25."Disabled and Grayed Out" ("Disabled")) -> ()  [unwired: 2 in, 2 out]
                  }
                }
                n641 = case shown="True" w1244 {
                  tunnel: w1243 -> [_ w1256]
                  tunnel: w1240 -> [_ w1255]
                  frame False {
                  }
                  frame True {
                    w1250 = enum16{"READ", "WRITE"}."WRITE" ("Action")
                    n642 = Decrement(x=w1256) -> (x-1=w1254:enum32{"Seq 1", "Seq 2", "Seq 3", "Seq 4"})
                    n643 = Index Array(array=w1255, index=w1254) -> (element=w1249:T40)
                    n644 = property on="Sequence List" class="RadioBtnsControl (strict)"("Value"=w1254) -> ()  [unwired: 2 in, 2 out]
                    n645 = Unbundle By Name(w1249) -> ("Detectors Parameters Out"=w1253:T17, "Laser Parameters Out"=w1252:T18, "Image Acquisition Parameters Out"=w1251:T19)
                    n646 = call "Detectors Crl_AE.vi"("Action"=w1250, "Detectors Parameters In"=w1253) -> ()  [unwired: 9 in, 1 out]
                    n647 = call "LASERs_ Crl_AE.vi"("Action"=w1250, "Laser Parameters In"=w1252) -> ()  [unwired: 9 in, 1 out]
                    n648 = call "Image Aquisition Param Ctrl_AE.vi"("Action"=w1250, "Image Acquisition Parameters In"=w1251) -> ()  [unwired: 9 in, 1 out]
                  }
                }
              }
            }
          }
          frame "DeleteAllSeq" {
            n649 = call "Seq AE.vi"("Action"=enum16{"READ", "BUILD", "WRITE", "DELETE"}."READ") -> ("Array"=w1258:T39)  [unwired: 8 in]
            n650 = Array Size(array=w1258) -> (size(s)=w1257:i32)
            n651 = flat-sequence {
              tunnel: w1257 -> [w1260]
              frame #0 {
                n652 = for {
                  N: w1260 -> [_]
                  n653 = call "Seq AE.vi"("Action"=enum16{"READ", "BUILD", "WRITE", "DELETE"}."DELETE") -> ()  [unwired: 8 in, 1 out]
                }
              }
              frame #1 {
                n654 = property on="Sequence List" class="RadioBtnsControl (strict)"("DisabledEnum"=T25."Disabled and Grayed Out" ("Disabled")) -> ()  [unwired: 2 in, 2 out]
              }
            }
          }
        }
      }
      event "Exit": Value Change {
        n655 = event-data() -> ("CtlRef"=w1287:refnum<vi>, "NewVal"=w1289:bool)  [unwired: 1 in, 1 out]
        n656 = Release Notifier(notifier=w1282, force destroy? (F)=TRUE) -> ()  [unwired: 1 in, 3 out]
        n657 = property class="Bool"(reference=w1287) -> ("Label.Text"=w1286:string)  [unwired: 1 in, 2 out]
        n658 = call "SLM AE.vi"("Action"=enum16{"READ", "WRITE"}."READ") -> ("SLM Ref Out"=w1280:refnum<vi>)  [unwired: 10 in]
        n659 = call "DM_Ref_AE.vi"("Action"=enum16{"READ", "WRITE"}."READ") -> ("DM Ref Out"=w1278:refnum<vi>)  [unwired: 10 in]
        n660 = call "GateDelay AE.vi"("Action"=enum16{"READ", "WRITE"}."READ") -> ("Gate Delay Ref Out"=w1279:refnum<vi>)  [unwired: 10 in]
        n661 = Enqueue Element(queue=w1288, element=w1286) -> ()  [unwired: 2 in, 3 out]
        n662 = Build Array(w1280, w1278, w1279) -> (w1277:refnum<vi>[])
        n663 = call "Stage_position_ae.vi"("StageID"="N664", "Enum"=enum16{"WRITE", "READ", "HOME", "SAVE HOME"}."HOME") -> ("Position Out"=w1269:dbl[])  [unwired: 8 in, 1 out]
        n664 = call "Stage_position_ae.vi"("StageID"="P541", "Enum"=enum16{"WRITE", "READ", "HOME", "SAVE HOME"}."HOME") -> ("Position Out"=w1273:dbl[])  [unwired: 8 in, 1 out]
        n665 = for {
          tunnel: w1277 -> [w1294] mode=indexing
          n666 = Not A Number/Path/Refnum?(number/path/refnum=w1294) -> (NaN/Path/Refnum?=w1293:bool)
          n667 = case shown="False" w1293 {
            tunnel: w1294 -> [w1295 _]
            frame False {
              n668 = To Variant(anything=TRUE) -> (Variant=w1296:variant)
              n669 = invoke class="VI" method="Ctrl Val.Set"(reference=w1295, "Control Name"="Exit", "Value"=w1296) -> (reference out=w1299:refnum<vi>)  [unwired: 2 in, 4 out]
              n670 = Close Reference(reference=w1299) -> ()  [unwired: 1 in, 1 out]
            }
            frame True {
            }
          }
        }
        n671 = Index Array(array=w1269, index=0) -> (element=w1266:dbl)
        n672 = property on="Stages" class="Clust (strict)"() -> ("Controls[]"=w1276:refnum<vi>[])  [unwired: 2 in, 2 out]
        n673 = Index Array(array=w1273, index=0) -> (element=w1267:dbl)
        n674 = Build Array(w1267, w1266) -> (w1265:dbl[])
        n675 = for {
          tunnel: w1276 -> [w1292] mode=indexing
          n676 = property class="Ctl"(reference=w1292) -> ("Label.Text"=w1291:string)  [unwired: 1 in, 2 out]
          n677 = call "All_Stages_Aloha.vi"("Aloha"=FALSE, "Stage ID"=w1291) -> ()  [unwired: 9 in, 1 out]
        }
        n678 = call-poly <vilib>:"Write To Spreadsheet File.vi"("format (%.3f)"="%.4f", "1D data"=w1265, "file path (dialog if empty)"=path "C:/Users/ED STED/Documents/Test Control Software/Host VIs/Stages/Stage Positions/home position.csv") -> ()  [unwired: 5 in, 1 out]
      }
    }
  }
  n679 = call "Manual Controls Action Engine.vi"("Action"=enum16{"Read", "Write"}."Write", "Manual Controls In"=w27) -> ("Manual Controls Out"=w29:T21)  [unwired: 13 in]
  n680 = call "FPGA-7842R-Control V2.vi"("Action"=FPGA-7842R-Reference."Initialize", "Manual Controls"=w29, "Initialize"=FALSE) -> ("Initalized"=w11:bool)  [unwired: 11 in, 1 out]
  n681 = while {
    shift-right: [w1312] -> _
    shift-left: "Idle" -> [w1313]
    tunnel: w18 -> [w1309]
    shift-right: [w1307] -> _
    shift-left: w11 -> [w1308]
    tunnel: w1 -> [w1300]
    stop <- w1311 stop-if-true
    n682 = call "Image Aquisition Param Ctrl_AE.vi"("Action"=enum16{"READ", "WRITE"}."READ") -> ("Image Acquisition Parameters Out"=w1306:T19)  [unwired: 10 in]
    n683 = call "Detectors Crl_AE.vi"("Action"=enum16{"READ", "WRITE"}."READ") -> ("Detectors Parameters Out"=w1304:T17)  [unwired: 10 in]
    n684 = call "Manual Controls Action Engine.vi"("Action"=enum16{"Read", "Write"}."Read") -> ("Manual Controls Out"=w1301:T21)  [unwired: 14 in]
    n685 = case shown="\"Display\"" w1313 {
      selector: w1313 -> [_ _ _ w1335 _ _ _ _ _ _]
      tunnel: ["Exit" w1322 "Idle" ("name (unnamed)") "Arange Displays" ("name (unnamed)") "Start FPGA Acquisition" ("name (unnamed)") "Display" ("name (unnamed)") "Close Images" ("name (unnamed)") "Idle" "Stop Waveforms" ("name (unnamed)") "Start Waveforms" ("name (unnamed)")] -> w1312
      tunnel: [TRUE w1324 w1331 w1342 w1411 w1437 w1478 w1511 w1520 w1558] -> w1311
      tunnel: FALSE -> [_ w1324 w1331 w1342 w1411 w1437 w1478 w1511 w1520 w1558]
      tunnel: w1309 -> [_ w1323 _ _ _ _ _ _ _ _]
      tunnel: w1308 -> [w1318 w1321 w1332 w1337 w1408 w1435 w1476 w1509 w1512 w1559]
      tunnel: [w1317 w1321 w1332 w1336 w1408 w1431 w1476 w1508 w1512 w1559] -> w1307
      tunnel: w1306 -> [_ _ _ w1340 _ w1430 _ _ _ w1556]
      tunnel: w1304 -> [_ _ _ w1339 _ _ _ _ _ w1554]
      tunnel: w1301 -> [_ _ _ w1338 _ _ _ _ _ _]
      tunnel: w1300 -> [_ _ _ _ w1401 _ _ _ _ _]
      frame "Exit" {
        n686 = call "Graph Ref AE.vi"("Action"=enum16{"READ", "WRITE"}."READ") -> ("Graph Ref Out"=w1315:refnum<vi>[])  [unwired: 10 in]
        n687 = call "FPGA-7842R-Control V2.vi"("Action"=FPGA-7842R-Reference."Close FPGA", "Initialize"=w1318) -> ("Initalized"=w1317:bool)  [unwired: 12 in, 1 out]
        n688 = Close Reference(reference=w1315) -> ()  [unwired: 1 in, 1 out]
      }
      frame "Idle", Default {
        n689 = Dequeue Element(queue=w1323, timeout in ms (-1)=-1) -> (element=w1322:string)  [unwired: 1 in, 3 out]
      }
      frame "Close Images" {
        w1327 = u16 0 items=["Read", "Write"] ("Mode")
        w1328 = u16 0 items=["Write", "Read"] ("Mode")
        n690 = call "File Action V1.vi"("Mode"=w1327) -> ("Files Open"=w1326:bool)  [unwired: 12 in, 2 out]
        n691 = call "Image_Actions_V1.vi"("Mode"=w1328, "Action"="Trash Images") -> ()  [unwired: 12 in, 2 out]
        n692 = case shown="True" w1326 {
          frame False {
          }
          frame True {
            w1334 = u16 1 items=["Read", "Write"] ("Mode")
            n693 = call "File Action V1.vi"("Action"="Close Files", "Mode"=w1334) -> ()  [unwired: 11 in, 3 out]
          }
        }
      }
      frame "Capture", "Live", "Sequence" {
        n694 = case shown="\"Live\", Default" w1335 {
          tunnel: w1340 -> [w1358 w1379 w1395]
          tunnel: w1339 -> [w1357 w1378 w1394]
          tunnel: w1338 -> [w1348 w1369 _]
          tunnel: w1337 -> [w1347 w1368 w1385]
          tunnel: [w1347 w1368 w1385] -> w1336
          frame "Capture" {
            w1345 = u16 1 items=["Read", "Write"] ("Mode")
            w1362 = u16 0 items=["Write", "Read"] ("Mode")
            n695 = Cluster To Array(cluster=w1357) -> (array=w1355:bool[])
            n696 = Index Array(array=w1355, index=4) -> (element=w1352:bool)
            n697 = Boolean To (0,1)(Boolean=w1355) -> (0, 1=w1356:i16[])
            n698 = Add Array Elements(numeric array=w1356) -> (sum=w1353:i16)
            n699 = To Long Integer(number=w1353) -> (32bit integer=w1350:i32)
            n700 = Unbundle By Name(w1358) -> ("Image Format"=w1359:u16)
            n701 = Select(t=1, s=w1352, f=w1350) -> (s? t:f=w1349:i32)
            n702 = call "File Action V1.vi"("Action"="Open Files", "Mode"=w1345, "Image Acquisition Parameters"=w1358, "Manual Controls In"=w1348, "File Path IN"="Save File Path", "Number of Channels"=w1349) -> ("File Path OUT"=w1343:path)  [unwired: 7 in, 2 out]
            n703 = local write "Save File Path"(w1343) -> ()
            n704 = To Long Integer(number=w1359) -> (32bit integer=w1361:i32)
            n705 = Bundle(w1361, w1361) -> (w1360:cluster{i32, i32})  [unwired: 1 in]
            n706 = call "Image_Actions_V1.vi"("Image Size (Pixels)"=w1360, "Mode"=w1362, "Number of Channels"=w1349, "Action"="Create Images") -> ()  [unwired: 10 in, 2 out]
          }
          frame "Sequence" {
            w1366 = u16 1 items=["Read", "Write"] ("Mode")
            w1383 = u16 0 items=["Write", "Read"] ("Mode")
            n707 = local read "Save File Path"() -> (w1365:path)
            n708 = Cluster To Array(cluster=w1378) -> (array=w1376:bool[])
            n709 = Index Array(array=w1376, index=4) -> (element=w1373:bool)
            n710 = Boolean To (0,1)(Boolean=w1376) -> (0, 1=w1377:i16[])
            n711 = Add Array Elements(numeric array=w1377) -> (sum=w1374:i16)
            n712 = To Long Integer(number=w1374) -> (32bit integer=w1371:i32)
            n713 = Unbundle By Name(w1379) -> ("Image Format"=w1380:u16)
            n714 = Select(t=1, s=w1373, f=w1371) -> (s? t:f=w1370:i32)
            n715 = call "File Action V1.vi"("Action"="Open Files", "Mode"=w1366, "Image Acquisition Parameters"=w1379, "Manual Controls In"=w1369, "File Path IN"=w1365, "Number of Channels"=w1370) -> ("File Path OUT"=w1364:path)  [unwired: 7 in, 2 out]
            n716 = local write "Save File Path"(w1364) -> ()
            n717 = To Long Integer(number=w1380) -> (32bit integer=w1382:i32)
            n718 = Bundle(w1382, w1382) -> (w1381:cluster{i32, i32})  [unwired: 1 in]
            n719 = call "Image_Actions_V1.vi"("Image Size (Pixels)"=w1381, "Mode"=w1383, "Number of Channels"=w1370, "Action"="Create Images") -> ()  [unwired: 10 in, 2 out]
          }
          frame "Live", Default {
            w1399 = u16 0 items=["Write", "Read"] ("Mode")
            n720 = Cluster To Array(cluster=w1394) -> (array=w1392:bool[])
            n721 = Index Array(array=w1392, index=4) -> (element=w1389:bool)
            n722 = Boolean To (0,1)(Boolean=w1392) -> (0, 1=w1393:i16[])
            n723 = Add Array Elements(numeric array=w1393) -> (sum=w1390:i16)
            n724 = To Long Integer(number=w1390) -> (32bit integer=w1387:i32)
            n725 = Unbundle By Name(w1395) -> ("Image Format"=w1396:u16)
            n726 = Select(t=1, s=w1389, f=w1387) -> (s? t:f=w1386:i32)
            n727 = To Long Integer(number=w1396) -> (32bit integer=w1398:i32)
            n728 = Bundle(w1398, w1398) -> (w1397:cluster{i32, i32})  [unwired: 1 in]
            n729 = call "Image_Actions_V1.vi"("Image Size (Pixels)"=w1397, "Mode"=w1399, "Number of Channels"=w1386, "Action"="Create Images") -> ()  [unwired: 10 in, 2 out]
          }
        }
      }
      frame "Arange Displays" {
        w1406 = u16 1 items=["Write", "Read"] ("Mode")
        w1409 = u16 1 items=["Read", "Write"] ("Action")
        n730 = call "Image_Actions_V1.vi"("Mode"=w1406) -> ("Image REFs OUT"=w1407:T49[])  [unwired: 13 in, 1 out]
        n731 = call "Graph Ref AE.vi"("Action"=enum16{"READ", "WRITE"}."READ", "Graph Ref In"=w1401) -> ("Graph Ref Out"=w1403:refnum<vi>[])  [unwired: 9 in]
        n732 = Array Size(array=w1407) -> (size(s)=w1405:i32)
        n733 = call "Arange_Displays_V2.vi"("Display References"=w1403, "Action"=w1409, "Number of Channels"=w1405, "Aspect Ratio (h/w)"=1.0) -> ("Number of Channels OUT"=w1404:i32)  [unwired: 11 in]
        n734 = for {
          N: w1404 -> [_]
          tunnel: w1403 -> [w1413] mode=indexing
          tunnel: [w1416] -> _ mode=indexing
          i -> [w1414]
          n735 = property class="IntGraph (strict)"(reference=w1413) -> ("Label.Text"=w1418:string)  [unwired: 1 in, 2 out]
          n736 = Equal To 0?(x=w1414) -> (x = 0?=w1415:bool)
          n737 = case shown="True" w1415 {
            tunnel: w1413 -> [_ w1419]
            frame False {
            }
            frame True {
              n738 = property class="IntGraph (strict)"(reference=w1419, "ZScale.Visible"=TRUE ("Z Scale.Visible"), "ZScale.Position"=T31 {"Left"=2431, "Top"=-320} ("Z Scale.Position")) -> ()  [unwired: 1 in, 2 out]
            }
          }
          n739 = To Unsigned Word Integer(number=w1414) -> (unsigned 16bit integer=w1417:u16)
          n740 = Bundle("Label.Text"=w1418, w1417) -> (w1416:cluster{"Label.Text":string, u16})  [unwired: 1 in]
        }
        "Graph Ref Out" <- w1401
      }
      frame "Start Waveforms" {
        n741 = call "Galvo Offset AE v1.vi"("Action"=enum16{"Read", "Write"}."Read") -> ("Galvo 1 Offset Out"=w1422:dbl)  [unwired: 1 in, 1 out]
        n742 = Unbundle By Name("Laser Controls 2") -> ("Laser On Time (Ticks)"=w1425:i8, "Laser Delay (Ticks)"=w1424:i8)
        n743 = call "Initialize Waveforms V4.vi"("Image Acquisition Parameters"=w1430, "Yale Galvo 1 Offset (V)"=w1422) -> ("Waveform Data to FPGA"=w1436:T50)  [unwired: 13 in]
        n744 = Unbundle By Name(w1430) -> ("Scan Type"=w1429:enum16{"Sample Scanning", "Beam Scanning"})
        n745 = call "FPGA-7842R-Control V2.vi"("Waveform Data"=w1436, "Action"=FPGA-7842R-Reference."Start Waveforms", "Laser On Time (Ticks)"=w1425, "Image Acquisition Parameters"=w1430, "Initialize"=w1435, "Laser Delay (Ticks)"=w1424) -> ("Initalized"=w1432:bool)  [unwired: 8 in, 1 out]
        n746 = Equal?(x=w1429, y=enum16{"Sample Scanning", "Beam Scanning"}."Sample Scanning" ("Scan Type")) -> (x = y?=w1427:bool)
        n747 = case shown="True" w1427 {
          tunnel: w1432 -> [w1438 w1443]
          tunnel: [w1438 w1442] -> w1431
          frame False {
          }
          frame True {
            n748 = call "Scan Parameters Action Engine.vi"("Action"=enum16{"Read", "Write"}."Read") -> ("Scan Parameters OUT"=w1440:T20)  [unwired: 14 in]
            n749 = Unbundle By Name(w1440) -> ("Unused_Axis_I16"=w1439:i16)
            n750 = call "FPGA-7842R-Control V2.vi"("Action"=FPGA-7842R-Reference."Unused Axis I16", "Initialize"=w1443, "Unused Axis Offset (I16)"=w1439) -> ("Initalized"=w1442:bool)  [unwired: 11 in, 1 out]
          }
        }
      }
      frame "Display" {
        w1471 = u16 1 items=["Write", "Read"] ("Mode")
        n751 = call "Image_Actions_V1.vi"("Mode"=w1471) -> ("Image REFs OUT"=w1473:T49[])  [unwired: 13 in, 1 out]
        n752 = Array Size(array=w1473) -> (size(s)=w1469:i32)
        n753 = Decrement(x=w1469) -> (x-1=w1468:i32)
        n754 = for {
          N: 6 -> [_]
          tunnel: w1468 -> [w1506]
          tunnel: [w1504] -> w1472 mode=indexing
          i -> [w1505]
          n755 = Greater Or Equal?(x=w1506, y=w1505) -> (x >= y?=w1504:bool)
        }
        n756 = Obtain Notifier(name (unnamed)="Running", notification data type=FALSE) -> (notifier out=w1445:refnum<notifier>)  [unwired: 2 in, 2 out]
        n757 = Index Array(array=w1472, index #1=1 ("index"), index #2=2 ("index"), index #3=3 ("index"), index #4=4 ("index"), index #5=5 ("index")) -> (element #1=w1457:bool, element #2=w1456:bool, element #3=w1455:bool, element #4=w1454:bool, element #5=w1453:bool)
        n758 = Index Array(array=w1473, index #1=0 ("index"), index #2=1 ("index"), index #3=2 ("index"), index #4=3 ("index"), index #5=4 ("index"), index #6=5 ("index")) -> (element #1=w1452:T49, element #2=w1451:T49, element #3=w1450:T49, element #4=w1449:T49, element #5=w1448:T49, element #6=w1447:T49)
        n759 = while {
          tunnel: w1457 -> [w1493]
          tunnel: w1456 -> [w1492]
          tunnel: w1455 -> [w1488]
          tunnel: w1454 -> [w1485]
          tunnel: w1453 -> [w1484]
          tunnel: w1452 -> [w1491]
          tunnel: w1451 -> [w1490]
          tunnel: w1450 -> [w1489]
          tunnel: w1449 -> [w1487]
          tunnel: w1448 -> [w1483]
          tunnel: w1447 -> [w1486]
          tunnel: w1445 -> [w1480]
          stop <- w1481 stop-if-true
          n760 = Get Notifier Status(notifier=w1480) -> (current notification=w1481:bool)  [unwired: 1 in, 4 out]
          n761 = case shown="True" w1493 {
            tunnel: w1490 -> [_ w1503]
            frame False {
            }
            frame True {
              n762 = call "IMAQ ImageToArray"("Image"=w1503) -> ("Image Pixels (Float)"=→"Channel 2":sgl[][])  [unwired: 3 in, 4 out]
            }
          }
          n763 = case shown="True" w1492 {
            tunnel: w1489 -> [_ w1501]
            frame False {
            }
            frame True {
              n764 = call "IMAQ ImageToArray"("Image"=w1501) -> ("Image Pixels (Float)"=→"Channel 3":sgl[][])  [unwired: 3 in, 4 out]
            }
          }
          n765 = call "IMAQ ImageToArray"("Image"=w1491) -> ("Image Pixels (Float)"=→"Channel 1":sgl[][])  [unwired: 3 in, 4 out]
          n766 = case shown="True" w1484 {
            tunnel: w1486 -> [_ w1495]
            frame False {
            }
            frame True {
              n767 = call "IMAQ ImageToArray"("Image"=w1495) -> ("Image Pixels (Float)"=→"Channel 6":sgl[][])  [unwired: 3 in, 4 out]
            }
          }
          n768 = case shown="True" w1485 {
            tunnel: w1483 -> [_ w1497]
            frame False {
            }
            frame True {
              n769 = call "IMAQ ImageToArray"("Image"=w1497) -> ("Image Pixels (Float)"=→"Channel 5":sgl[][])  [unwired: 3 in, 4 out]
            }
          }
          n770 = case shown="True" w1488 {
            tunnel: w1487 -> [_ w1499]
            frame False {
            }
            frame True {
              n771 = call "IMAQ ImageToArray"("Image"=w1499) -> ("Image Pixels (Float)"=→"Channel 4":sgl[][])  [unwired: 3 in, 4 out]
            }
          }
          n772 = Wait (ms)(milliseconds to wait=u32 100) -> ()  [unwired: 1 out]
        }
      }
      frame "Stop Waveforms" {
        n773 = call "FPGA-7842R-Control V2.vi"("Action"=FPGA-7842R-Reference."Stop Waveforms", "Initialize"=w1509) -> ("Initalized"=w1508:bool)  [unwired: 12 in, 1 out]
      }
      frame "Stop Acquisition" {
        n774 = call "FPGA-7842R-Control V2.vi"("Action"=FPGA-7842R-Reference."Laser Control", "Laser Controls"=T18 {"STED Power (V)"=0.0, "STED"=FALSE, "650 nm"=FALSE, "590 nm"=FALSE, "485 nm"=FALSE, "Manual Control"=FALSE} ("Laser Controls 2"), "Initialize"=TRUE) -> ()  [unwired: 11 in, 2 out]
        n775 = call "AO AE.vi"("Action"=enum16{"READ", "WRITE"}."READ") -> ("Z Comp. Output"=w1514:T1)  [unwired: 8 in, 2 out]
        n776 = Unbundle By Name(w1514) -> ("Enable"=w1513:bool)
        n777 = case shown="True" w1513 {
          frame False {
          }
          frame True {
            n778 = call "Image Aquisition Param Ctrl_AE.vi"("Action"=enum16{"READ", "WRITE"}."READ") -> ("Image Acquisition Parameters Out"=w1524:T19)  [unwired: 10 in]
            n779 = Unbundle By Name(w1524) -> ("Scan Mode"=w1523:enum16{"XY", "XZ", "YZ", "XYZ"})
            n780 = Equal?(x=w1523, y=enum16{"XY", "XZ", "YZ", "XYZ"}."XYZ") -> (x = y?=w1521:bool)
            n781 = case shown="False" w1521 {
              frame False {
              }
              frame True {
                w1528 = 1 ("disabled index (col)")
                w1530 = 0 ("disabled index (col)")
                n782 = call "AO AE.vi"("Action"=enum16{"READ", "WRITE"}."READ") -> ("Mirror Modes Out"=w1532:T38, "DM Value Output"=w1535:dbl[][], "Z Comp. Output"=w1546:T1)  [unwired: 8 in]
                n783 = call "Mirror_Mode_DUAL_AE.vi"("Action"=Standard_Action."Write", "Mirror Modes In"=w1532) -> ()  [unwired: 13 in, 1 out]
                n784 = call "Deform_Mirror_DUAL_AE_V2.vi"("Action"=Standard_Action."Read") -> ("Refnum Out"=w1540:refnum<k7>, "Multi Map Data Out"=w1538:i32[])  [unwired: 10 in, 3 out]
                n785 = Index Array(array=w1535, index (col)=w1530) -> (element=w1531:dbl[])  [unwired: 1 in]
                n786 = Unbundle By Name(w1546) -> ("Origin (um)"=w1549:dbl)
                n787 = call "Voltage vs Signal_Data Engine_V1.vi"("Control Signal In (-1~1)"=w1531, "DM #"=w1530) -> ("Voltage Out (0~Max. Vol.)"=w1529:dbl[])  [unwired: 1 in, 1 out]
                n788 = control-ref of="Abort AllStage"() -> (w1542:refnum<vi>)
                n789 = call "WriteDM_V2.vi"("reference in"=w1540, "nDevId"=0, "MultiDM  Mapping"=w1538, "Voltage Array in"=w1529) -> ("reference out"=w1539:refnum<k7>)  [unwired: 2 in, 1 out]
                n790 = Build Array(w1549) -> (w1548:dbl[])
                n791 = Bundle By Name(cluster=w1546, "Enable"=FALSE) -> (w1544:T1)
                n792 = Index Array(array=w1535, index (col)=w1528) -> (element=w1527:dbl[])  [unwired: 1 in]
                n793 = call "AE_AllStages_Action V2.vi"("Velocity"=10000.0, "Abort"=w1542, "Positions"=w1548, "Axis"=bool[] [TRUE], "Stage ID"="P841", "Action"=StageStates."MOVE") -> ()  [unwired: 3 in, 3 out]
                n794 = call "Voltage vs Signal_Data Engine_V1.vi"("Control Signal In (-1~1)"=w1527, "DM #"=w1528) -> ("Voltage Out (0~Max. Vol.)"=w1526:dbl[])  [unwired: 1 in, 1 out]
                n795 = call "WriteDM_V2.vi"("reference in"=w1539, "nDevId"=1, "MultiDM  Mapping"=w1538, "Voltage Array in"=w1526) -> ()  [unwired: 2 in, 2 out]
                n796 = call "AO AE.vi"("Mirror Modes In"=w1532, "DM Value Input"=w1535, "Z Comp. Input"=w1544, "Action"=enum16{"READ", "WRITE"}."WRITE") -> ()  [unwired: 5 in, 3 out]
                n797 = call "Pixel Value (-1 to 1) DUAL AE.vi"("Action"=Standard_Action."Write", "Pixel Value (-1 to 1)"=w1535) -> ()  [unwired: 13 in, 1 out]
              }
            }
          }
        }
      }
      frame "Start FPGA Acquisition" {
        n798 = Unbundle By Name(w1556) -> ("Scan Mode"=w1555:enum16{"XY", "XZ", "YZ", "XYZ"})
        n799 = case shown="\"XZ\", Default" w1555 {
          tunnel: w1556 -> [_ w1567]
          tunnel: w1554 -> [_ w1566]
          frame "YZ" {
            n800 = vi-ref "FPGA Sample Scanning V1.vi"() -> (w1562:refnum<vi>)
            n801 = property class="VI Interface Type 4"(reference=w1562) -> ("Path"=w1560:path)  [unwired: 1 in, 2 out]
            n802 = Open VI Reference(type specifier VI Refnum (for type only)=w1562, vi path=w1560, options=128) -> (vi reference=w1563:refnum<vi>)  [unwired: 3 in, 1 out]
            n803 = call-by-ref "Start Asynchronous Call"(reference=w1563) -> (reference out=w1564:refnum<vi>)  [unwired: 4 in, 1 out]
            n804 = Close Reference(reference=w1564) -> ()  [unwired: 1 in, 1 out]
          }
          frame "XZ", Default {
            n805 = vi-ref "FPGA Beam Scanning V2.vi"() -> (w1569:refnum<vi>)
            n806 = property class="VI Interface Type 5"(reference=w1569) -> ("Path"=w1570:path)  [unwired: 1 in, 2 out]
            n807 = Open VI Reference(type specifier VI Refnum (for type only)=w1569, vi path=w1570, options=128) -> (vi reference=w1568:refnum<vi>)  [unwired: 3 in, 1 out]
            n808 = call-by-ref "Start Asynchronous Call"(reference=w1568, "Detectors"=w1566, "Image Acquisition Parameters"=w1567) -> (reference out=w1565:refnum<vi>)  [unwired: 3 in, 1 out]
            n809 = Close Reference(reference=w1565) -> ()  [unwired: 1 in, 1 out]
          }
        }
      }
    }
  }
